vi "JKI_Controller.vi"() -> ()   [LabVIEW 2017, in "Controller_JKI.lvlib"]
uses:
  Controller_JKI.lvlib
  Transaction.ctl
  <userlib>/_NEVSTOP/JKI State Machine ++/_Support/_Create Data Queue.vi
  <userlib>/_NEVSTOP/JKI State Machine ++/_Support/_JKISMQFGV.vi
  <userlib>/_OpenG.lib/array/array.llb/Search 1D Array (String)__ogtk.vi
  <userlib>/_NEVSTOP/JKI State Machine ++/JKI-State-Machine-Plus.lvlib
panel:
  in  "Log In Init Simulator":bool
  out "State History":string
  in  "Name(\"\" to use uuid)":string="Controller"
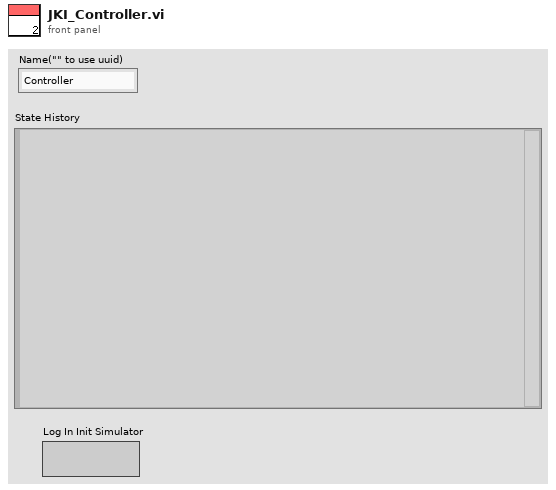
[diagram p1: front panel]
types:
  T1 = typedef "Controller_JKI.lvlib/Transaction.ctl" = enum16{"Welcome", "Login", "Idle ", "Invalid Login", "Terminate Session", "Deposit", "Withdrawl", "Fast Cash", "Withdrawl Complete", "Withdrawl Failed", "Balance Inquiry"}
  T2 = enum32{"Invalid", "Standard", "Closed", "Hidden", "Minimized", "Maximized"}
  T3 = enum32{"invalid app kind", "Development System", "Run Time System", "Student Edition", "Embedded LabVIEW", "Evaluation", "Custom"}
  T4 = cluster{"Core":cluster{"Current VI Reference":refnum<vi>, "Close Panel on Exit?":bool}, "Transactions":T1, "Log in attempts":i32, "First":string, "Last":string, "PIN":string, "Amount":i32, "Money":i32}
  T5 = cluster{"Current VI Reference":refnum<vi>, "Close Panel on Exit?":bool}
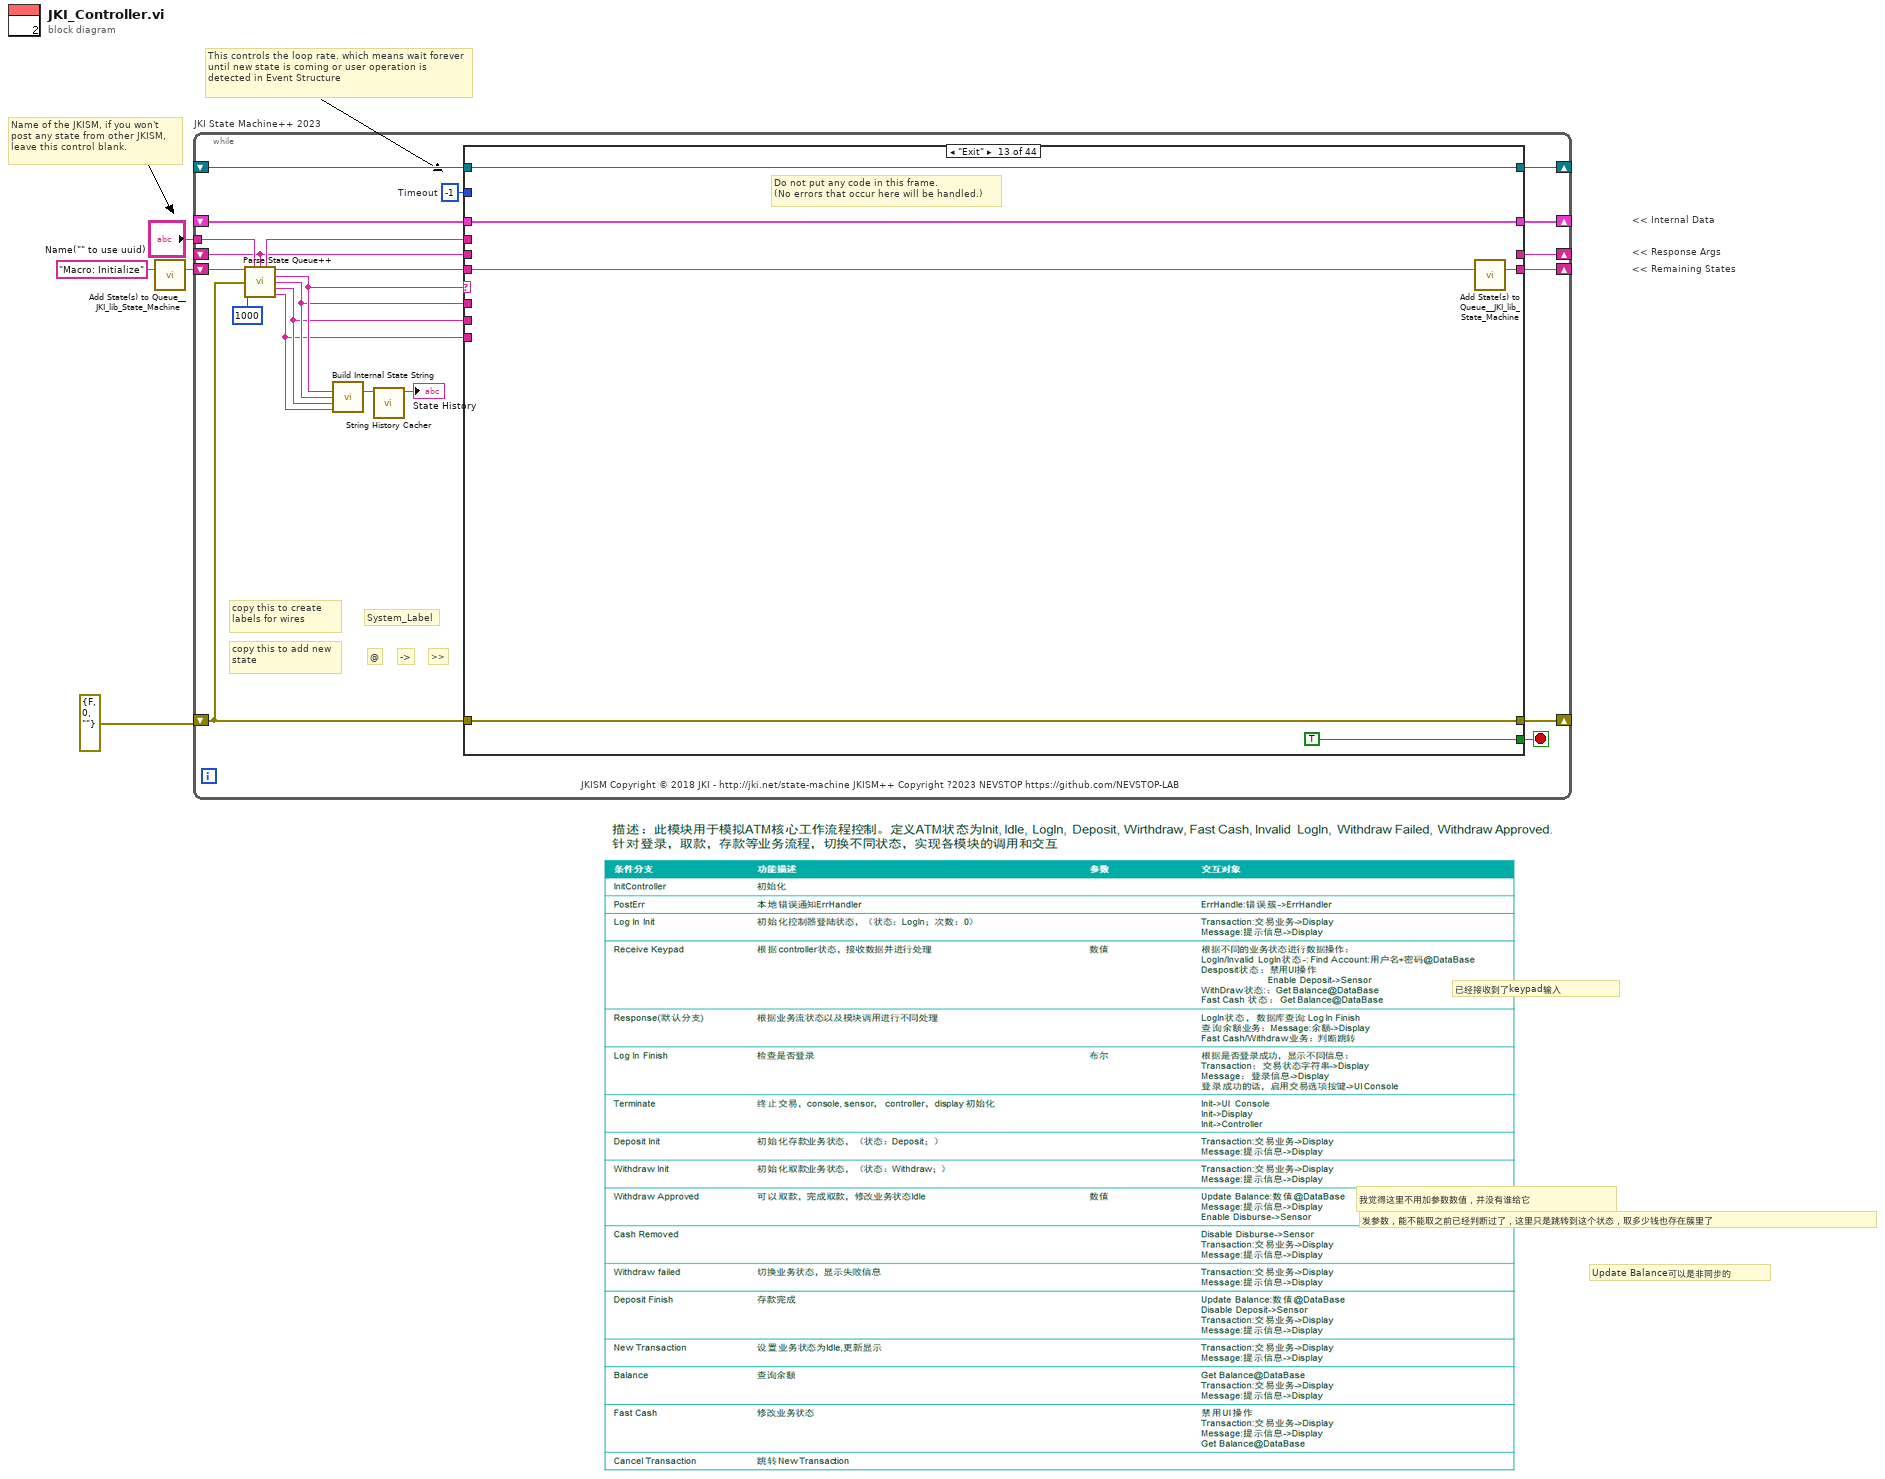
[diagram p0: block diagram]
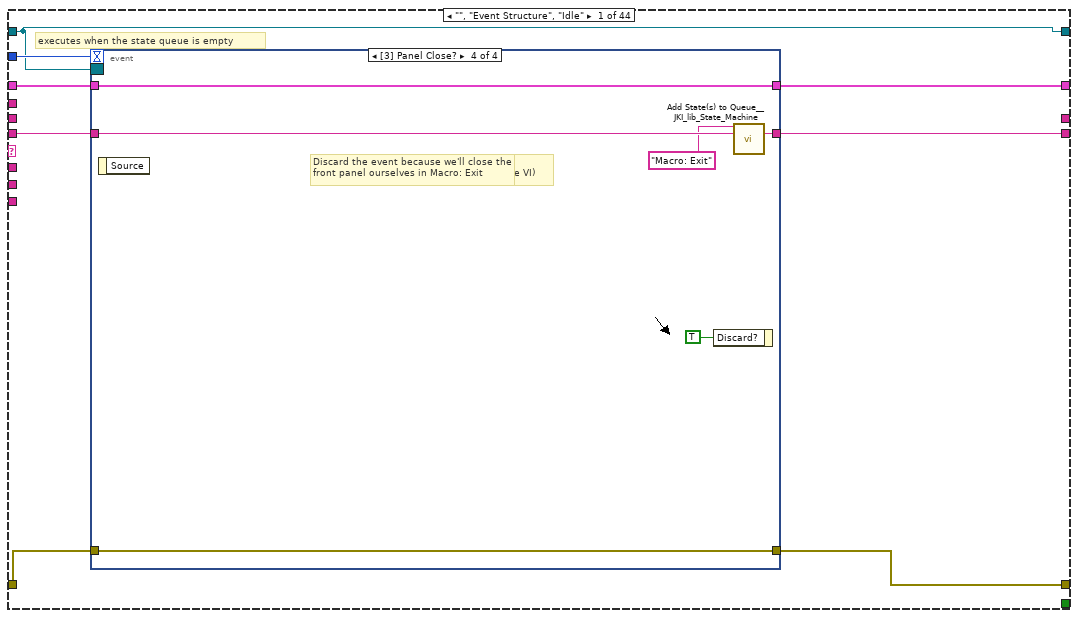
[diagram p2: hidden frame]
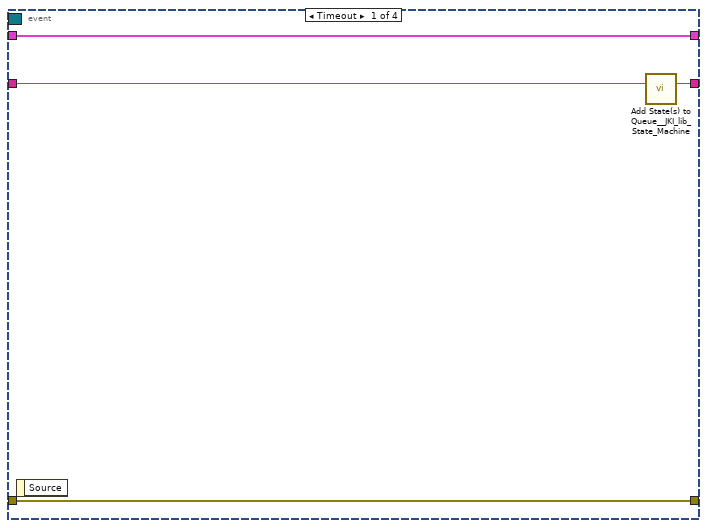
[diagram p3: hidden frame]
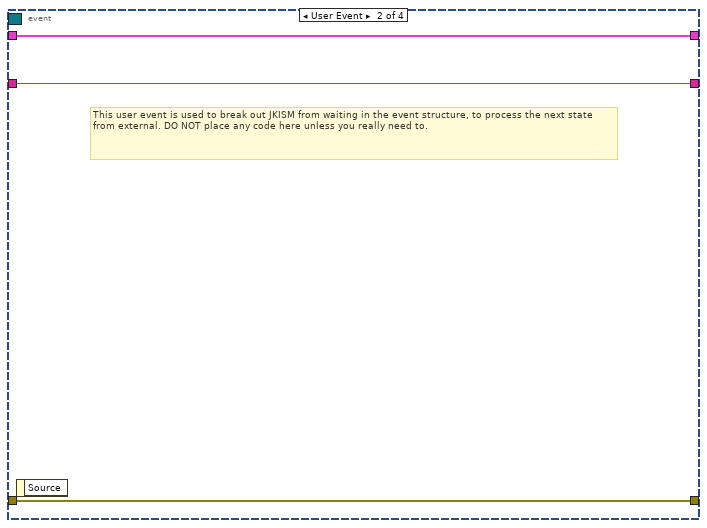
[diagram p4: hidden frame]
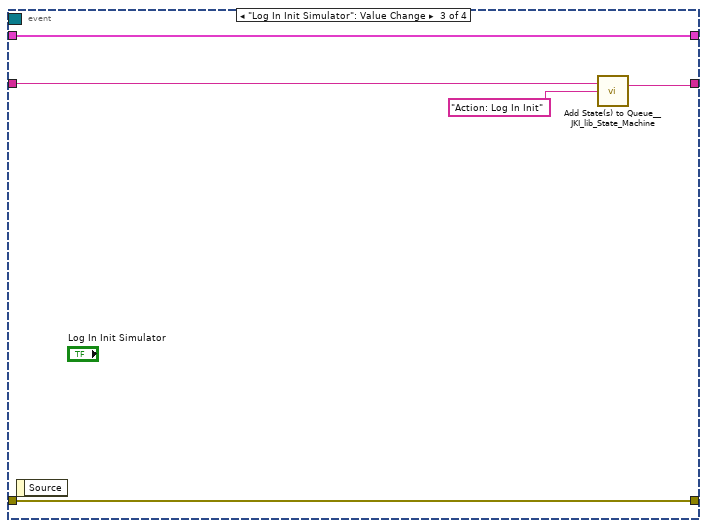
[diagram p5: hidden frame]
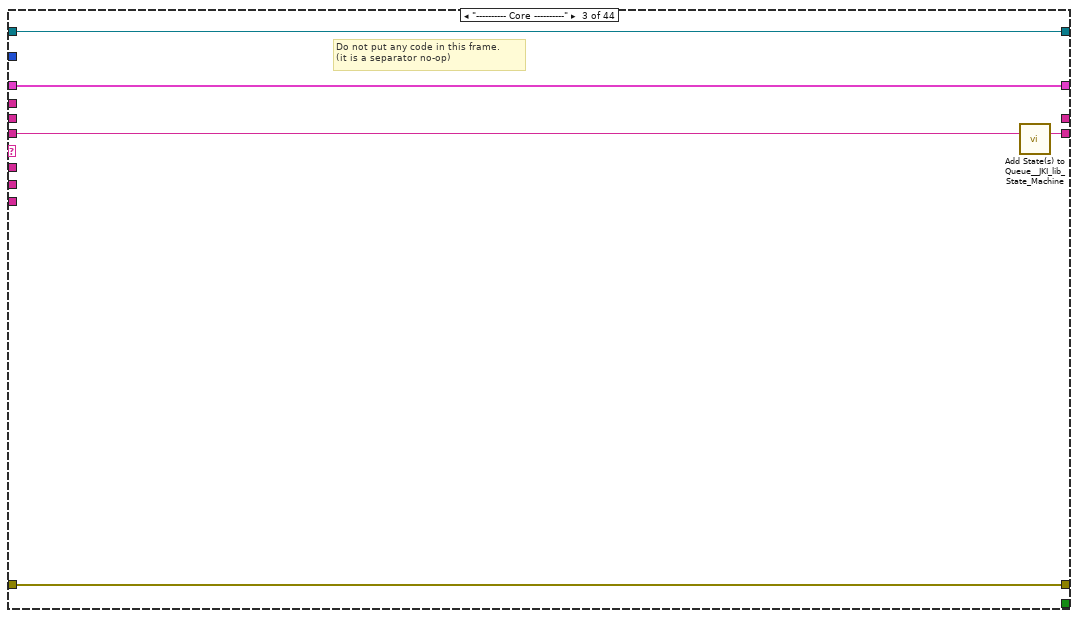
[diagram p7: hidden frame]
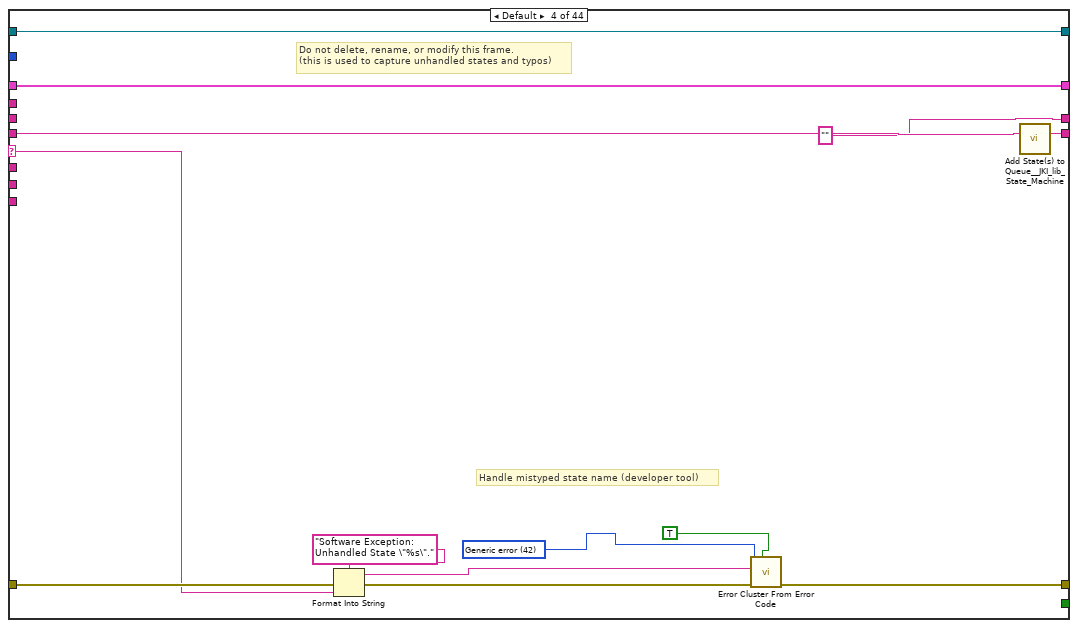
[diagram p8: hidden frame]
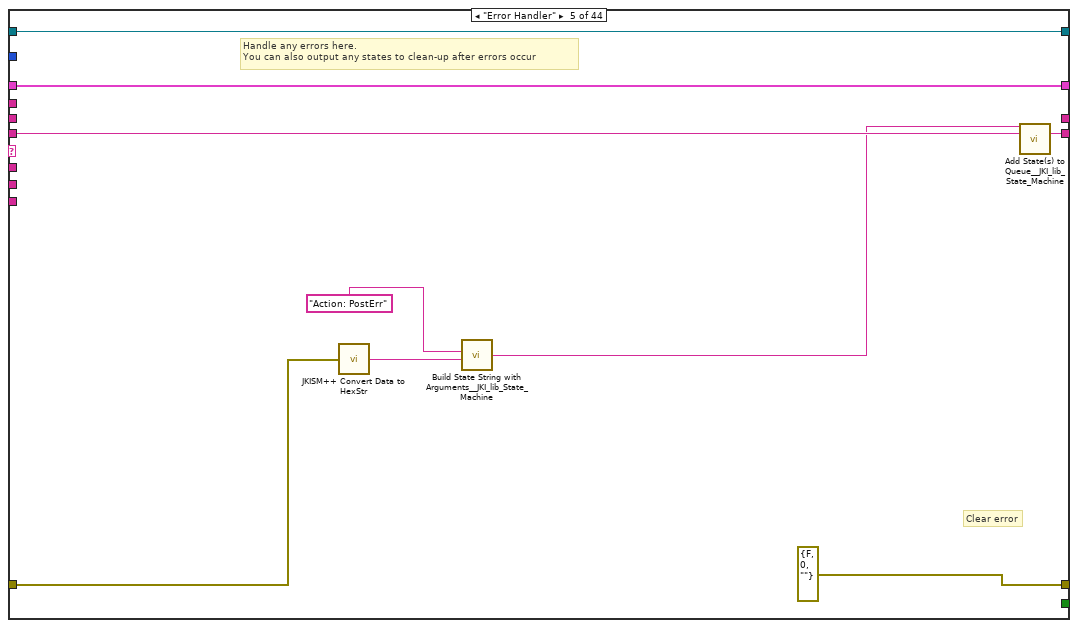
[diagram p9: hidden frame]
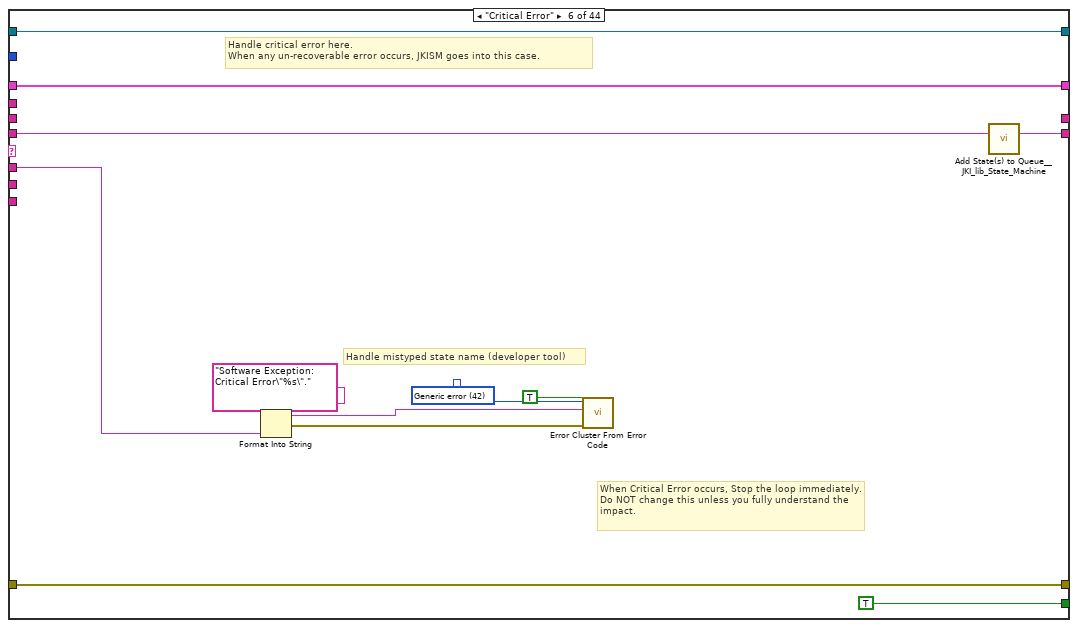
[diagram p10: hidden frame]
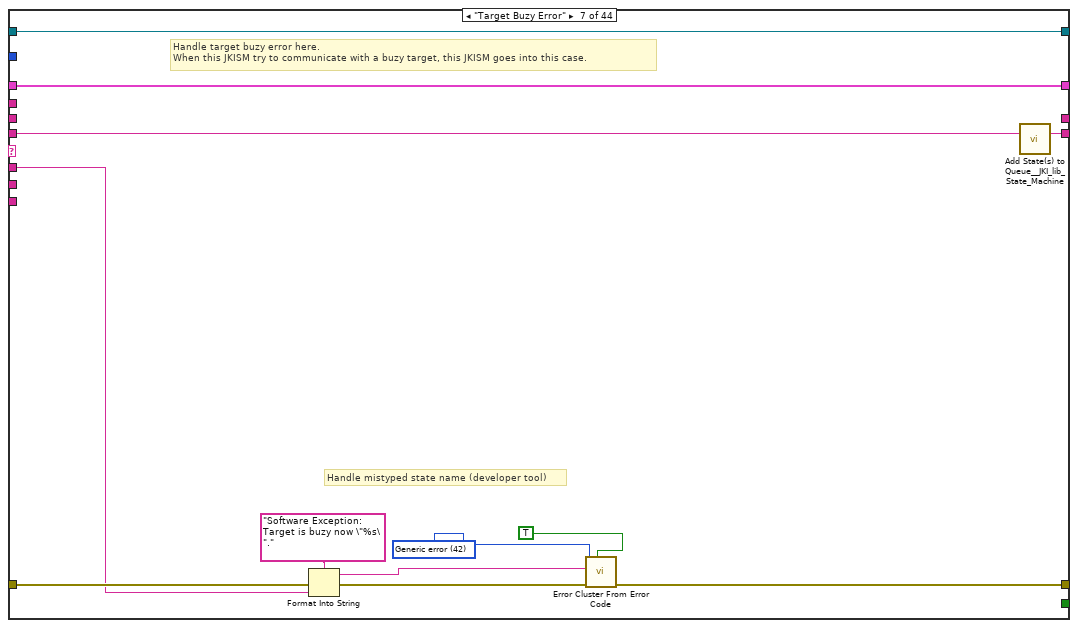
[diagram p11: hidden frame]
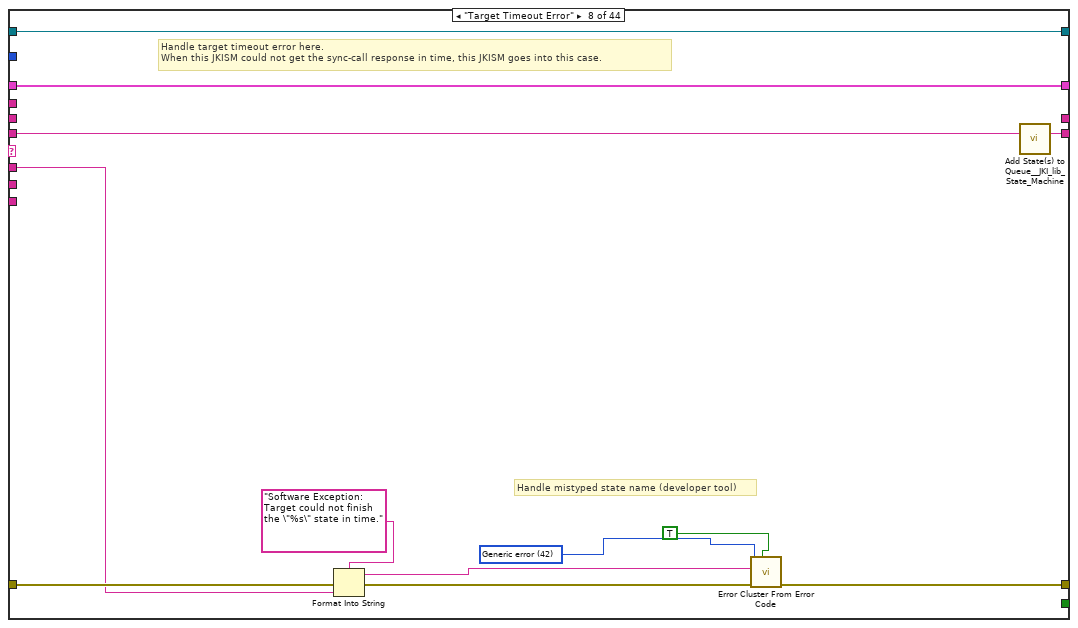
[diagram p12: hidden frame]
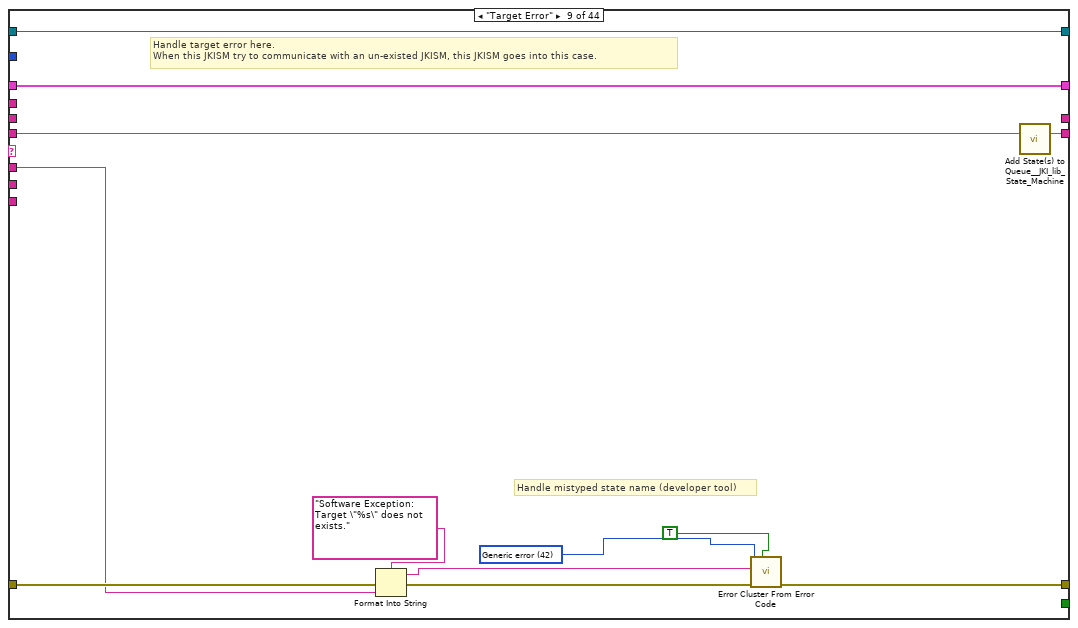
[diagram p13: hidden frame]
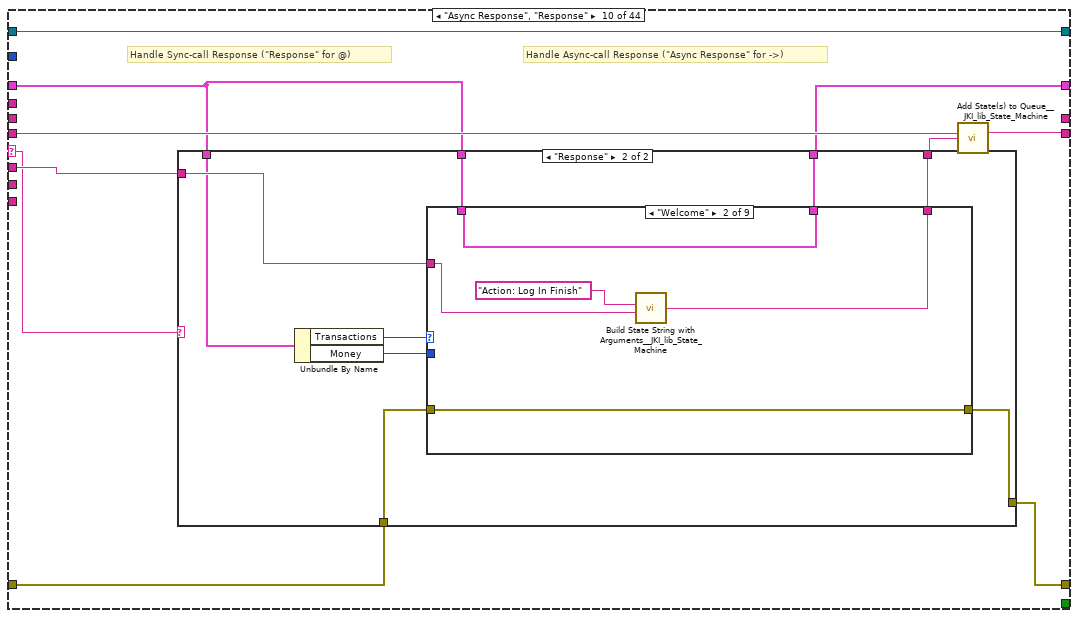
[diagram p14: hidden frame]
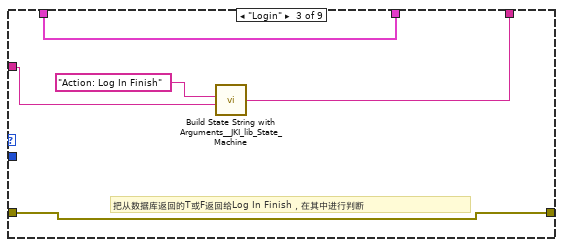
[diagram p17: hidden frame]
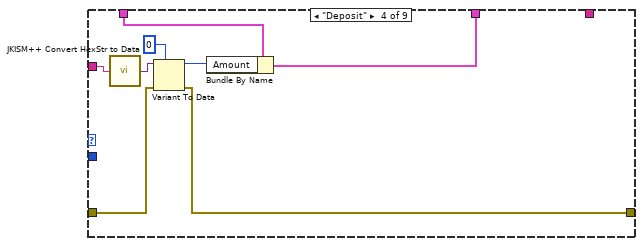
[diagram p18: hidden frame]
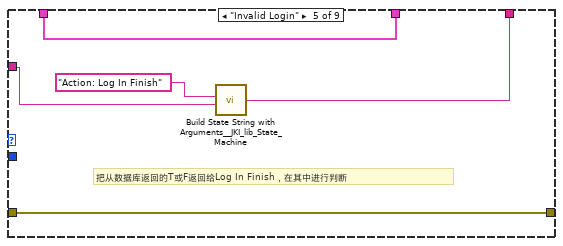
[diagram p19: hidden frame]
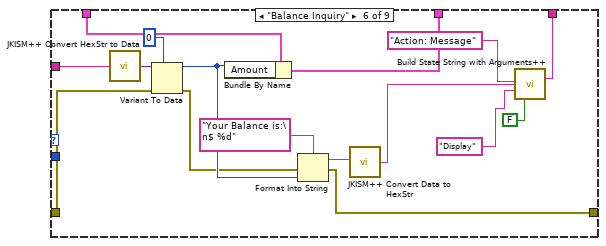
[diagram p20: hidden frame]
diagram:
  # "Update Balance可以是非同步的"
  # "发参数，能不能取之前已经判断过了，这里只是跳转到这个状态，取多少钱也存在簇里了"
  # "我觉得这里不用加参数数值，并没有谁给它"
  # "已经接收到了keypad输入"
  # "<< Internal Data"
  # "<< Response Args"
  # "<< Remaining States"
  # "Name of the JKISM, if you won't post any state from other JKISM,  leave this control blank."
  # "This controls the loop rate. which means wait forever until new state is coming or user operation is detected in Event Structure"
  n1 = call <vilib>:"Add State(s) to Queue__JKI_lib_State_Machine.vi"("State(s) in (\"\")"="Macro: Initialize") -> ("States Out"=w2:string)  [unwired: 14 in]
  n2 = while "JKI State Machine++ 2023" {
    shift-right: [w21] -> _
    shift-left: _ -> [w20]
    shift-right: [w24] -> _
    shift-left: errorcluster {"status"=FALSE, "code"=0, "source"=""} ("error in (no error)") -> [w18]
    shift-right: [w23] -> _
    shift-left: w2 -> [w25]
    tunnel: "Name(\"\" to use uuid)" -> [w13]
    shift-right: [w16] -> _
    shift-left: _ -> [w5]
    shift-right: [w15] -> _
    shift-left: _ -> [w14]
    stop <- w22 stop-if-true
    w19 = -1  # Timeout
    # "JKISM Copyright © 2018 JKI - http://jki.net/state-machine JKISM++ Copyright ?2023 NEVSTOP https://github.com/NEVSTOP-LAB"
    # "copy this to add new state"
    # ">>"
    # "->"
    # "@"
    # "copy this to create labels for wires"
    # "System_Label"
    n3 = call <userlib>:"Parse State Queue++.vi"("State Queue"=w25, "Name(\"\" to use uuid)"=w13, "Response Arguments"=w5, "Error In (no error)"=w18, "Response Timeout(5000ms)"=1000 ("Response Timeout(1000ms)")) -> ("Name Used"=w6:string, "Remaining States"=w26:string, "Current State"=w10:string, "Arguments"=w9:string, "Argument - State"=w8:string, "From Who"=w7:string)  [unwired: 5 in]
    n4 = call <userlib>:"Build Internal State String.vi"("State"=w10, "Arguments (\"\")"=w9, "Arg-State (\"\")"=w8, "Source (\"\")"=w7) -> ("State with Arguments"=w11:string)  [unwired: 11 in]
    n5 = call <userlib>:"String History Cacher.vi"("String"=w11) -> ("String Cache"=→"State History":string)  [unwired: 10 in]
    n6 = case shown="\"Exit\"" w10 {
      selector: w10 -> [_ _ _ w64 _ _ _ _ _ w133 _ _ _ _ _ _ _ _ _ _ _ _ _ _ _ _ _ _ _ _ _ _ _ _ _ _ _ _ _ _ _ _ _ _]
      tunnel: w26 -> [w34 w55 w61 w68 w83 w93 w96 w113 w125 w139 w255 w270 w276 w281 w294 w301 w306 w312 w316 w322 w327 w334 w346 w416 w422 w444 w467 w476 w479 w505 w521 w619 w691 w707 w725 w759 w792 w815 w846 w881 w899 w946 w952 w967]
      tunnel: w9 -> [_ _ _ _ _ w86 w98 w109 w121 w140 _ _ _ _ _ _ _ _ _ _ _ w329 w340 _ _ _ _ _ _ w489 w528 w626 _ _ _ _ _ _ _ _ _ _ _ _]
      tunnel: w20 -> [w32 w54 w58 w66 w80 w94 w100 w111 w123 w132 w254 w263 w274 w278 _ w296 w303 w311 w315 w319 w325 w332 w342 w413 w419 w442 w466 w472 w484 w517 w527 w615 w693 w701 w720 w773 w786 w810 w871 w878 w896 w928 w954 w964]
      tunnel: [w31 w56 w59 w70 errorcluster {"status"=FALSE, "code"=0, "source"=""} ("error out") w95 w103 w115 w127 w135 w256 w267 w273 w279 w291 w297 w304 w307 w314 w320 w324 w330 w343 w414 w420 w427 w468 w474 w485 w497 w522 w616 w679 w704 w723 w740 w796 w813 w830 w876 w894 w919 w961 w965] -> w24
      tunnel: w18 -> [w30 w56 w59 w69 w76 w95 w102 w114 w126 w137 w256 w267 w273 w279 w291 w298 w304 _ w317 w320 w324 w331 w344 w414 w420 w434 w468 w474 w485 w498 w522 w622 w679 w704 w723 w741 w796 w813 w831 w876 w894 w919 w961 w965]
      tunnel: [w33 w55 w60 w67 w82 w92 w101 w112 w124 w138 w255 w269 w275 w280 w293 w300 w305 w312 w316 w321 w326 w333 w345 w415 w421 w443 w467 w475 w478 w504 w520 w618 w690 w706 w726 w758 w791 w816 w845 w880 w898 w945 w951 w966] -> w23
      tunnel: [_ _ _ _ _ TRUE _ _ _ _ _ _ TRUE _ _ _ _ _ _ _ _ _ _ _ _ _ _ _ _ _ _ _ _ _ _ _ _ _ _ _ _ _ _ _] -> w22
      tunnel: [w29 w54 w58 w66 w80 w94 w100 w111 w123 w136 w254 w268 w274 w278 w292 w296 w303 w311 w315 w319 w325 w332 w342 w413 w419 w442 w466 w470 w484 w515 w526 w614 w693 w698 w719 w772 w785 w808 w870 w877 w895 w927 w955 w964] -> w21
      tunnel: w19 -> [w28 _ _ _ _ _ _ _ _ _ _ _ _ _ _ _ _ _ _ _ _ _ _ _ _ _ _ _ _ _ _ _ _ _ _ _ _ _ _ _ _ _ _ _]
      tunnel: w7 -> [_ _ _ _ _ _ _ _ _ _ _ _ _ _ _ _ _ _ _ _ _ _ _ _ _ _ _ _ _ _ _ _ _ _ _ _ _ _ _ _ _ _ _ _]
      tunnel: w8 -> [_ _ _ _ _ _ _ _ _ _ _ _ _ _ _ _ _ _ _ _ _ _ _ _ _ _ _ _ _ _ _ _ _ _ _ _ _ _ _ _ _ _ _ _]
      tunnel: [_ _ _ "" _ _ _ _ _ _ _ _ _ _ _ _ _ _ _ _ _ _ _ _ _ _ _ _ _ _ _ _ _ _ _ _ _ _ _ _ _ _ _ _] -> w16
      tunnel: [w27 w53 w57 w62 w79 w84 w97 w108 w120 w141 w253 w257 w271 w277 w289 w295 w302 w310 w313 w318 w323 w328 w339 w412 w417 w436 w465 w473 w483 w518 w531 w627 w692 w717 w737 w775 w807 w827 w872 w892 w910 w949 w960 w963] -> w15
      tunnel: w14 -> [w27 w53 w57 w62 w79 w84 w97 w108 w120 w141 w253 w257 w271 w277 w289 w295 w302 _ w313 w318 w323 w328 w339 w412 w417 w436 w465 w473 w483 w518 w531 w627 w692 w717 w737 w775 w807 w827 w872 w892 w910 w949 w960 w963]
      tunnel: w6 -> [_ _ _ _ _ _ _ _ _ _ _ _ _ _ _ _ _ w309 _ _ _ _ _ _ _ _ _ _ _ _ _ _ _ _ _ _ _ _ _ _ _ _ _ _]
      tunnel: w5 -> [_ _ _ _ _ _ _ _ _ _ _ _ _ _ _ _ _ _ _ _ _ _ _ _ _ _ _ _ _ _ _ _ _ _ _ _ _ _ _ _ _ _ _ _]
      frame "", "Event Structure", "Idle" {
        # "executes when the state queue is empty"
        n7 = event shown="[3] Panel Close?" {
          selector: w27 -> [_ _ _ _]
          dyn-events: _ -> [_ _ _ _]
          timeout: w28 -> [_ _ _ _]
          tunnel: w34 -> [w38 w40 w44 w52]
          tunnel: [w37 w40 w43 w51] -> w33
          tunnel: w32 -> [w35 w41 w45 w49]
          tunnel: [w36 w39 w46 w50] -> w31
          tunnel: w30 -> [w36 w39 w46 w50]
          tunnel: [w35 w41 w45 w49] -> w29
          event Timeout {
            n8 = event-data() -> ()  [unwired: 1 in, 1 out]
            n9 = call <vilib>:"Add State(s) to Queue__JKI_lib_State_Machine.vi"("State(s) in (\"\")"=w38) -> ("States Out"=w37:string)  [unwired: 14 in]
          }
          event User Event {
            # "This user event is used to break out JKISM from waiting in the event structure, to process the next state from external. DO NOT place any code here unless you really need to."
            n10 = event-data() -> ()  [unwired: 1 in, 1 out]
          }
          event "Log In Init Simulator": Value Change {
            n11 = event-data() -> ()  [unwired: 1 in, 1 out]
            n12 = call <vilib>:"Add State(s) to Queue__JKI_lib_State_Machine.vi"("State(s) in (\"\")"=w44, "State(s) at Back (\"\")"="Action: Log In Init" ("State(s) at Back (\"\")")) -> ("States Out"=w43:string)  [unwired: 13 in]
          }
          event Panel Close? {
            # "Discard the event because we'll close the front panel ourselves in Macro: Exit"
            # "Close Panel button (pressed) Event\n(this executes Macro: Exit to terminate the VI)"
            n13 = event-data() -> ()  [unwired: 1 in, 1 out]
            n14 = event-data("Discard?"=TRUE) -> ()  [unwired: 1 in, 1 out]
            n15 = call <vilib>:"Add State(s) to Queue__JKI_lib_State_Machine.vi"("State(s) in Front (\"\")"="Macro: Exit", "State(s) in (\"\")"=w52) -> ("States Out"=w51:string)  [unwired: 13 in]
          }
        }
      }
      frame "JKISM++ Documentation" {
        # "JKISM++ Documentation"
        # "State Syntax:\nStateCategory: State >> Argument @|-> JKISMName\nLine Terminator: Line feed\n\nExample:\nUI: Help >> About @Main\nUI: Help >> About ->Main"
        # "Commenting:\nTo add a comment use \"//\" or \"#\" and all text to the right will be ignored\nCommenting Example:\nUI: Initialize // This initializes the UI\n# This whole line is a comment\n// Another comment line"
        # "Where \"UI\" is the state category\nWhere \"Help\" is the state\nWhere \"About\" is the argument\nWhere \"Main\" is the Name of JKISM,which actually run the \"UI: Help >> About\"\n\n    \"@\" stands for sync state. Current JKISM will wait until the state is finished. \n            - if \"Main\" named JKISM does not exist, \"Target Error\" will occur.\n            - if \"Main\" named JKISM is in another sync remote state, \"Target Buzy Error\" will occur.\n            - if \"Main\" named JKISM could not finish the state in time, \"Target Timeout Error\" will occur.\n            - if everything is right. \"Response\" will occur with Argument back from \"Main\" named JKISM. \n\n    \"->\" stands for async state. Current JKISM will post the state and continue to next state in next iteration.\n            - if \"Main\" named JKISM does not exist, \"Target Error\" will occur.\n            - if everything is right. \"Async Message Posted\" will occur.\n            - After State is finished. Caller will receive a \"Async Response\" state from callee.\n\nWhen duplicated name is used for multiple JKISM module or some framework problem happens, \"Critical Error\" will occur."
      }
      frame "---------- Core ----------" {
        # "Do not put any code in this frame.\n(it is a separator no-op)"
        n16 = call <vilib>:"Add State(s) to Queue__JKI_lib_State_Machine.vi"("State(s) in (\"\")"=w61) -> ("States Out"=w60:string)  [unwired: 14 in]
      }
      frame Default {
        w73 = 42 items=["No error", "Argument error", "Memory is full", "Out of zone", "End of file", "File already open", "Generic file I/O error", "File not found", "File permission error", "Disk is full", "Duplicate path", "Too many files open", "System feature not enabled", "Resource file not found", "Cannot add resource", "Resource not found", "Image not found", "Image memory error", "Pen does not exist", "Config type invalid", "Config token not found", "Config parse error", "Config memory error", "Bad external code format", "Bad external code offset", "External code not present", "Null window", "Destroy window error", "Null menu", "Print aborted", "Bad print record", "Print driver error", "Windows error during printing", "Memory error during printing", "Print dialog error", "Generic print error", "Invalid device refnum", "Device not found", "Device parameter error", "Device unit error", "Cannot open device", "Device call aborted", "Generic error", "Cancelled by user", "Object ID too low", "Object ID too high", "Object not in heap", "Unknown heap", "Unknown object (invalid DefProc)", "Unknown object (DefProc not in table)", "Message out of range", "Invalid (null) method", "Unknown message", "Manager call not supported", "Bad address", "Network operation in progress", "Network operation timed out", "Connection is busy", "Network attribute not supported", "Network error", "Address in use", "System out of memory", "Connection aborted", "Connection refused", "Not connected", "Already connected", "Connection closed", "Initialization error (interapplication manager)", "Bad occurrence", "Wait on unbound occurrence handler", "Occurrence queue overflow", "Datalog type conflict", "Unused", "Unrecognized type (interapplication manager)", "Memory corrupt", "Failed to make temporary DLL", "Old CIN version", "Drag socket not found", "Failed to load drop-object", "Failed to register OLE object", "Failed to release OLE object", "Format specifier type mismatch", "Unknown format specifier", "Too few format specifiers", "Too many format specifiers", "Scan failed", "Newer CIN version", "Error converting to variant", "Runtime menu error", "Password tampered", "Variant attribute not found", "Incompatible variant data type", "Event data is not available", "Event Store is not present", "Occurrence is not found", "Event Queue is not created", "Event info is not available", "Refnum passed is NULL", "Error retrieving Class GUID", "Error retrieving CoClass GUID", "Error retrieving TypeLib GUID.", "Bad built application magic bytes.", "Specific driver is different from the specific driver associated with the Logical Name.", "There is no session opened to the class driver.", "Max Error", "MAX - Error with config objects", "MAX - Error loading configuration", "MAX - Group not supported"]
        # "Do not delete, rename, or modify this frame.\n(this is used to capture unhandled states and typos)"
        # "Handle mistyped state name (developer tool)"
        n17 = Format Into String(format string="Software Exception: Unhandled State \"%s\"." ("message"), error in=w69, w64) -> (resulting string=w72:string, error out=w71:errorcluster)  [unwired: 1 in]
        n18 = call <vilib>:"Error Cluster From Error Code.vi"("show call chain? (False)"=TRUE, "error in (no error)"=w71, "error message (\"\")"=w72, "error code (0)"=w73) -> ("error out"=w70:errorcluster)  [unwired: 5 in]
        n19 = call <vilib>:"Add State(s) to Queue__JKI_lib_State_Machine.vi"("State(s) in (\"\")"=w68) -> ("States Out"=w67:string)  [unwired: 14 in]
      }
      frame "Error Handler" {
        # "Handle any errors here.\nYou can also output any states to clean-up after errors occur"
        # "Clear error"
        n20 = call <userlib>:"JKISM++ Convert Data to HexStr.vi"("Variant"=w76) -> ("HEX String (0-9,A-F)"=w78:string)  [unwired: 8 in]
        n21 = call <vilib>:"Build State String with Arguments__JKI_lib_State_Machine.vi"("Arguments (\"\")"=w78, "State"="Action: PostErr") -> ("State with Arguments"=w75:string)  [unwired: 4 in]
        n22 = call <vilib>:"Add State(s) to Queue__JKI_lib_State_Machine.vi"("State(s) in Front (\"\")"=w75, "State(s) in (\"\")"=w83) -> ("States Out"=w82:string)  [unwired: 13 in]
      }
      frame "Critical Error" {
        w90 = 42 items=["No error", "Argument error", "Memory is full", "Out of zone", "End of file", "File already open", "Generic file I/O error", "File not found", "File permission error", "Disk is full", "Duplicate path", "Too many files open", "System feature not enabled", "Resource file not found", "Cannot add resource", "Resource not found", "Image not found", "Image memory error", "Pen does not exist", "Config type invalid", "Config token not found", "Config parse error", "Config memory error", "Bad external code format", "Bad external code offset", "External code not present", "Null window", "Destroy window error", "Null menu", "Print aborted", "Bad print record", "Print driver error", "Windows error during printing", "Memory error during printing", "Print dialog error", "Generic print error", "Invalid device refnum", "Device not found", "Device parameter error", "Device unit error", "Cannot open device", "Device call aborted", "Generic error", "Cancelled by user", "Object ID too low", "Object ID too high", "Object not in heap", "Unknown heap", "Unknown object (invalid DefProc)", "Unknown object (DefProc not in table)", "Message out of range", "Invalid (null) method", "Unknown message", "Manager call not supported", "Bad address", "Network operation in progress", "Network operation timed out", "Connection is busy", "Network attribute not supported", "Network error", "Address in use", "System out of memory", "Connection aborted", "Connection refused", "Not connected", "Already connected", "Connection closed", "Initialization error (interapplication manager)", "Bad occurrence", "Wait on unbound occurrence handler", "Occurrence queue overflow", "Datalog type conflict", "Unused", "Unrecognized type (interapplication manager)", "Memory corrupt", "Failed to make temporary DLL", "Old CIN version", "Drag socket not found", "Failed to load drop-object", "Failed to register OLE object", "Failed to release OLE object", "Format specifier type mismatch", "Unknown format specifier", "Too few format specifiers", "Too many format specifiers", "Scan failed", "Newer CIN version", "Error converting to variant", "Runtime menu error", "Password tampered", "Variant attribute not found", "Incompatible variant data type", "Event data is not available", "Event Store is not present", "Occurrence is not found", "Event Queue is not created", "Event info is not available", "Refnum passed is NULL", "Error retrieving Class GUID", "Error retrieving CoClass GUID", "Error retrieving TypeLib GUID.", "Bad built application magic bytes.", "Specific driver is different from the specific driver associated with the Logical Name.", "There is no session opened to the class driver.", "Max Error", "MAX - Error with config objects", "MAX - Error loading configuration", "MAX - Group not supported"]
        # "Handle critical error here.\nWhen any un-recoverable error occurs, JKISM goes into this case."
        # "When Critical Error occurs, Stop the loop immediately. Do NOT change this unless you fully understand the impact."
        # "Handle mistyped state name (developer tool)"
        n23 = Format Into String(format string="Software Exception: Critical Error\"%s\"." ("message"), w86) -> (resulting string=w89:string, error out=w88:errorcluster)  [unwired: 2 in]
        n24 = call <vilib>:"Error Cluster From Error Code.vi"("show call chain? (False)"=TRUE, "error in (no error)"=w88, "error message (\"\")"=w89, "error code (0)"=w90) -> ()  [unwired: 5 in, 1 out]
        n25 = call <vilib>:"Add State(s) to Queue__JKI_lib_State_Machine.vi"("State(s) in (\"\")"=w93) -> ("States Out"=w92:string)  [unwired: 14 in]
      }
      frame "Target Buzy Error" {
        w106 = 42 items=["No error", "Argument error", "Memory is full", "Out of zone", "End of file", "File already open", "Generic file I/O error", "File not found", "File permission error", "Disk is full", "Duplicate path", "Too many files open", "System feature not enabled", "Resource file not found", "Cannot add resource", "Resource not found", "Image not found", "Image memory error", "Pen does not exist", "Config type invalid", "Config token not found", "Config parse error", "Config memory error", "Bad external code format", "Bad external code offset", "External code not present", "Null window", "Destroy window error", "Null menu", "Print aborted", "Bad print record", "Print driver error", "Windows error during printing", "Memory error during printing", "Print dialog error", "Generic print error", "Invalid device refnum", "Device not found", "Device parameter error", "Device unit error", "Cannot open device", "Device call aborted", "Generic error", "Cancelled by user", "Object ID too low", "Object ID too high", "Object not in heap", "Unknown heap", "Unknown object (invalid DefProc)", "Unknown object (DefProc not in table)", "Message out of range", "Invalid (null) method", "Unknown message", "Manager call not supported", "Bad address", "Network operation in progress", "Network operation timed out", "Connection is busy", "Network attribute not supported", "Network error", "Address in use", "System out of memory", "Connection aborted", "Connection refused", "Not connected", "Already connected", "Connection closed", "Initialization error (interapplication manager)", "Bad occurrence", "Wait on unbound occurrence handler", "Occurrence queue overflow", "Datalog type conflict", "Unused", "Unrecognized type (interapplication manager)", "Memory corrupt", "Failed to make temporary DLL", "Old CIN version", "Drag socket not found", "Failed to load drop-object", "Failed to register OLE object", "Failed to release OLE object", "Format specifier type mismatch", "Unknown format specifier", "Too few format specifiers", "Too many format specifiers", "Scan failed", "Newer CIN version", "Error converting to variant", "Runtime menu error", "Password tampered", "Variant attribute not found", "Incompatible variant data type", "Event data is not available", "Event Store is not present", "Occurrence is not found", "Event Queue is not created", "Event info is not available", "Refnum passed is NULL", "Error retrieving Class GUID", "Error retrieving CoClass GUID", "Error retrieving TypeLib GUID.", "Bad built application magic bytes.", "Specific driver is different from the specific driver associated with the Logical Name.", "There is no session opened to the class driver.", "Max Error", "MAX - Error with config objects", "MAX - Error loading configuration", "MAX - Group not supported"]
        # "Handle target buzy error here.\nWhen this JKISM try to communicate with a buzy target, this JKISM goes into this case."
        # "Handle mistyped state name (developer tool)"
        n26 = Format Into String(format string="Software Exception: Target is buzy now \"%s\"." ("message"), error in=w102, w98) -> (resulting string=w105:string, error out=w104:errorcluster)  [unwired: 1 in]
        n27 = call <vilib>:"Error Cluster From Error Code.vi"("show call chain? (False)"=TRUE, "error in (no error)"=w104, "error message (\"\")"=w105, "error code (0)"=w106) -> ("error out"=w103:errorcluster)  [unwired: 5 in]
        n28 = call <vilib>:"Add State(s) to Queue__JKI_lib_State_Machine.vi"("State(s) in (\"\")"=w96) -> ("States Out"=w101:string)  [unwired: 14 in]
      }
      frame "Target Timeout Error" {
        w118 = 42 items=["No error", "Argument error", "Memory is full", "Out of zone", "End of file", "File already open", "Generic file I/O error", "File not found", "File permission error", "Disk is full", "Duplicate path", "Too many files open", "System feature not enabled", "Resource file not found", "Cannot add resource", "Resource not found", "Image not found", "Image memory error", "Pen does not exist", "Config type invalid", "Config token not found", "Config parse error", "Config memory error", "Bad external code format", "Bad external code offset", "External code not present", "Null window", "Destroy window error", "Null menu", "Print aborted", "Bad print record", "Print driver error", "Windows error during printing", "Memory error during printing", "Print dialog error", "Generic print error", "Invalid device refnum", "Device not found", "Device parameter error", "Device unit error", "Cannot open device", "Device call aborted", "Generic error", "Cancelled by user", "Object ID too low", "Object ID too high", "Object not in heap", "Unknown heap", "Unknown object (invalid DefProc)", "Unknown object (DefProc not in table)", "Message out of range", "Invalid (null) method", "Unknown message", "Manager call not supported", "Bad address", "Network operation in progress", "Network operation timed out", "Connection is busy", "Network attribute not supported", "Network error", "Address in use", "System out of memory", "Connection aborted", "Connection refused", "Not connected", "Already connected", "Connection closed", "Initialization error (interapplication manager)", "Bad occurrence", "Wait on unbound occurrence handler", "Occurrence queue overflow", "Datalog type conflict", "Unused", "Unrecognized type (interapplication manager)", "Memory corrupt", "Failed to make temporary DLL", "Old CIN version", "Drag socket not found", "Failed to load drop-object", "Failed to register OLE object", "Failed to release OLE object", "Format specifier type mismatch", "Unknown format specifier", "Too few format specifiers", "Too many format specifiers", "Scan failed", "Newer CIN version", "Error converting to variant", "Runtime menu error", "Password tampered", "Variant attribute not found", "Incompatible variant data type", "Event data is not available", "Event Store is not present", "Occurrence is not found", "Event Queue is not created", "Event info is not available", "Refnum passed is NULL", "Error retrieving Class GUID", "Error retrieving CoClass GUID", "Error retrieving TypeLib GUID.", "Bad built application magic bytes.", "Specific driver is different from the specific driver associated with the Logical Name.", "There is no session opened to the class driver.", "Max Error", "MAX - Error with config objects", "MAX - Error loading configuration", "MAX - Group not supported"]
        # "Handle target timeout error here.\nWhen this JKISM could not get the sync-call response in time, this JKISM goes into this case."
        # "Handle mistyped state name (developer tool)"
        n29 = Format Into String(format string="Software Exception: Target could not finish the \"%s\" state in time." ("message"), error in=w114, w109) -> (resulting string=w117:string, error out=w116:errorcluster)  [unwired: 1 in]
        n30 = call <vilib>:"Error Cluster From Error Code.vi"("show call chain? (False)"=TRUE, "error in (no error)"=w116, "error message (\"\")"=w117, "error code (0)"=w118) -> ("error out"=w115:errorcluster)  [unwired: 5 in]
        n31 = call <vilib>:"Add State(s) to Queue__JKI_lib_State_Machine.vi"("State(s) in (\"\")"=w113) -> ("States Out"=w112:string)  [unwired: 14 in]
      }
      frame "Target Error" {
        w130 = 42 items=["No error", "Argument error", "Memory is full", "Out of zone", "End of file", "File already open", "Generic file I/O error", "File not found", "File permission error", "Disk is full", "Duplicate path", "Too many files open", "System feature not enabled", "Resource file not found", "Cannot add resource", "Resource not found", "Image not found", "Image memory error", "Pen does not exist", "Config type invalid", "Config token not found", "Config parse error", "Config memory error", "Bad external code format", "Bad external code offset", "External code not present", "Null window", "Destroy window error", "Null menu", "Print aborted", "Bad print record", "Print driver error", "Windows error during printing", "Memory error during printing", "Print dialog error", "Generic print error", "Invalid device refnum", "Device not found", "Device parameter error", "Device unit error", "Cannot open device", "Device call aborted", "Generic error", "Cancelled by user", "Object ID too low", "Object ID too high", "Object not in heap", "Unknown heap", "Unknown object (invalid DefProc)", "Unknown object (DefProc not in table)", "Message out of range", "Invalid (null) method", "Unknown message", "Manager call not supported", "Bad address", "Network operation in progress", "Network operation timed out", "Connection is busy", "Network attribute not supported", "Network error", "Address in use", "System out of memory", "Connection aborted", "Connection refused", "Not connected", "Already connected", "Connection closed", "Initialization error (interapplication manager)", "Bad occurrence", "Wait on unbound occurrence handler", "Occurrence queue overflow", "Datalog type conflict", "Unused", "Unrecognized type (interapplication manager)", "Memory corrupt", "Failed to make temporary DLL", "Old CIN version", "Drag socket not found", "Failed to load drop-object", "Failed to register OLE object", "Failed to release OLE object", "Format specifier type mismatch", "Unknown format specifier", "Too few format specifiers", "Too many format specifiers", "Scan failed", "Newer CIN version", "Error converting to variant", "Runtime menu error", "Password tampered", "Variant attribute not found", "Incompatible variant data type", "Event data is not available", "Event Store is not present", "Occurrence is not found", "Event Queue is not created", "Event info is not available", "Refnum passed is NULL", "Error retrieving Class GUID", "Error retrieving CoClass GUID", "Error retrieving TypeLib GUID.", "Bad built application magic bytes.", "Specific driver is different from the specific driver associated with the Logical Name.", "There is no session opened to the class driver.", "Max Error", "MAX - Error with config objects", "MAX - Error loading configuration", "MAX - Group not supported"]
        # "Handle target error here.\nWhen this JKISM try to communicate with an un-existed JKISM, this JKISM goes into this case."
        # "Handle mistyped state name (developer tool)"
        n32 = Format Into String(format string="Software Exception: Target \"%s\" does not exists." ("message"), error in=w126, w121) -> (resulting string=w129:string, error out=w128:errorcluster)  [unwired: 1 in]
        n33 = call <vilib>:"Error Cluster From Error Code.vi"("show call chain? (False)"=TRUE, "error in (no error)"=w128, "error message (\"\")"=w129, "error code (0)"=w130) -> ("error out"=w127:errorcluster)  [unwired: 5 in]
        n34 = call <vilib>:"Add State(s) to Queue__JKI_lib_State_Machine.vi"("State(s) in (\"\")"=w125) -> ("States Out"=w124:string)  [unwired: 14 in]
      }
      frame "Async Response", "Response" {
        # "Handle Async-call Response (\"Async Response\" for ->)"
        # "Handle Sync-call Response (\"Response\" for @)"
        n35 = case shown="\"Response\"" w133 {
          tunnel: w140 -> [_ w151]
          tunnel: w137 -> [w142 w150]
          tunnel: w132 -> [w143 w149]
          tunnel: [w143 w148] -> w136
          tunnel: [w142 w147] -> w135
          tunnel: [_ w145] -> w134
          tunnel: w132 -> [_ w144]
          frame "Async Response", Default {
          }
          frame "Response" {
            n36 = Unbundle By Name(w149) -> ("Transactions"=w152:T1, "Money"=w146:i32)
            n37 = case shown="\"Welcome\"" w152 {
              tunnel: w151 -> [_ w157 w163 w169 w176 w191 w201 w220 w241]
              tunnel: [_ w156 w161 _ w174 w181 w202 w224 w244] -> w145
              tunnel: w150 -> [w153 w155 w160 w167 w173 w184 w198 w223 w234]
              tunnel: w144 -> [w154 w158 w164 w172 w177 w193 w196 w218 w239]
              tunnel: [w154 w158 w164 w171 w177 w192 w195 w217 w238] -> w148
              tunnel: [w153 w155 w160 w166 w173 w182 w197 w223 w233] -> w147
              tunnel: w146 -> [_ _ _ _ _ _ _ w215 w236]
              frame Default {
              }
              frame "Welcome" {
                n38 = call <vilib>:"Build State String with Arguments__JKI_lib_State_Machine.vi"("Arguments (\"\")"=w157, "State"="Action: Log In Finish") -> ("State with Arguments"=w156:string)  [unwired: 4 in]
              }
              frame "Login" {
                # "把从数据库返回的T或F返回给Log In Finish，在其中进行判断"
                n39 = call <vilib>:"Build State String with Arguments__JKI_lib_State_Machine.vi"("Arguments (\"\")"=w163, "State"="Action: Log In Finish") -> ("State with Arguments"=w161:string)  [unwired: 4 in]
              }
              frame "Deposit" {
                n40 = call <userlib>:"JKISM++ Convert HexStr to Data.vi"("HEX String"=w169) -> ("Variant"=w168:variant)  [unwired: 8 in]
                n41 = Variant To Data(error in=w167, type=0, Variant=w168) -> (data=w165:i32, error out=w166:errorcluster)
                n42 = Bundle By Name(cluster=w172, "Amount"=w165) -> (w171:T4)
              }
              frame "Invalid Login" {
                # "把从数据库返回的T或F返回给Log In Finish，在其中进行判断"
                n43 = call <vilib>:"Build State String with Arguments__JKI_lib_State_Machine.vi"("Arguments (\"\")"=w176, "State"="Action: Log In Finish") -> ("State with Arguments"=w174:string)  [unwired: 4 in]
              }
              frame "Balance Inquiry" {
                n44 = call <userlib>:"JKISM++ Convert HexStr to Data.vi"("HEX String"=w191) -> ("Variant"=w190:variant)  [unwired: 8 in]
                n45 = Variant To Data(error in=w184, type=0, Variant=w190) -> (data=w185:i32, error out=w183:errorcluster)
                n46 = Bundle By Name(cluster=w193, "Amount"=w185) -> (w192:T4)
                n47 = Format Into String(format string="Your Balance is:\n$ %d", error in=w183, w185) -> (resulting string=w179:string, error out=w182:errorcluster)  [unwired: 1 in]
                n48 = call <userlib>:"JKISM++ Convert Data to HexStr.vi"("Variant"=w179) -> ("HEX String (0-9,A-F)"=w178:string)  [unwired: 8 in]
                n49 = call <userlib>:"Build State String with Arguments++.vi"("State"="Action: Message" ("States"), "Arguments (\"\")"=w178, "Dest Module (\"\")"="Display" ("Dest Module"), "Sync-Call(@) T By Default/Async-Call(->) F"=FALSE) -> ("State with Arguments"=w181:string)  [unwired: 11 in]
              }
              frame "Fast Cash" {
                n50 = call <userlib>:"JKISM++ Convert HexStr to Data.vi"("HEX String"=w201) -> ("Variant"=w200:variant)  [unwired: 8 in]
                n51 = Variant To Data(error in=w198, type=0 ("y"), Variant=w200) -> (data=w194:i32, error out=w197:errorcluster)
                n52 = Greater Or Equal?(x=w194, y=50) -> (x >= y?=w203:bool)
                n53 = case shown="False" w203 {
                  tunnel: ["Action: Withdraw Failed" "Action: Fast Cash"] -> w202
                  tunnel: w196 -> [w208 w212]
                  tunnel: [w206 w210] -> w195
                  tunnel: w194 -> [_ w211]
                  frame False {
                    # "余额不足即把本次交易额归零"
                    n54 = Bundle By Name(cluster=w208, "Money"=0, "Transactions"=Transaction."Withdrawl Failed") -> (w206:T4)
                  }
                  frame True {
                    n55 = Bundle By Name(cluster=w212, "Amount"=w211) -> (w210:T4)
                  }
                }
              }
              frame "Withdrawl" {
                # "这里是keypad String"
                n56 = call <userlib>:"JKISM++ Convert HexStr to Data.vi"("HEX String"=w220) -> ("Variant"=w222:variant)  [unwired: 8 in]
                n57 = Variant To Data(type=0 ("y"), Variant=w222) -> (data=w216:i32)  [unwired: 1 in, 1 out]
                n58 = Negate(x=w215) -> (-x=w214:i32)
                n59 = Greater Or Equal?(x=w216, y=w214) -> (x >= y?=w219:bool)
                n60 = case shown="True" w219 {
                  tunnel: ["Action: Withdraw Failed" "Action: Withdraw Approved"] -> w224
                  tunnel: w218 -> [w227 w231]
                  tunnel: [w225 w229] -> w217
                  tunnel: w216 -> [_ w230]
                  frame False {
                    n61 = Bundle By Name(cluster=w227, "Money"=0) -> (w225:T4)
                  }
                  frame True {
                    n62 = Bundle By Name(cluster=w231, "Amount"=w230) -> (w229:T4)
                  }
                }
              }
              frame "Withdrawl Failed" {
                # "这里是keypad String"
                n63 = call <userlib>:"JKISM++ Convert HexStr to Data.vi"("HEX String"=w241) -> ("Variant"=w243:variant)  [unwired: 8 in]
                n64 = Variant To Data(error in=w234, type=0 ("y"), Variant=w243) -> (data=w237:i32, error out=w233:errorcluster)
                n65 = Negate(x=w236) -> (-x=w235:i32)
                n66 = Greater Or Equal?(x=w237, y=w235) -> (x >= y?=w240:bool)
                n67 = case shown="True" w240 {
                  tunnel: ["Action: Withdraw Failed" "Action: Withdraw Approved"] -> w244
                  tunnel: w239 -> [w247 w251]
                  tunnel: [w245 w249] -> w238
                  tunnel: w237 -> [_ w250]
                  frame False {
                    n68 = Bundle By Name(cluster=w247, "Money"=0) -> (w245:T4)
                  }
                  frame True {
                    n69 = Bundle By Name(cluster=w251, "Amount"=w250) -> (w249:T4)
                  }
                }
              }
            }
          }
        }
        n70 = call <vilib>:"Add State(s) to Queue__JKI_lib_State_Machine.vi"("State(s) in (\"\")"=w139, "State(s) at Back (\"\")"=w134) -> ("States Out"=w138:string)  [unwired: 13 in]
      }
      frame "Async Message Posted" {
        # "Handle post action for async message (->)."
        # "After Async Message is posted (->), JKISM+ goes to this state for post-action. You can use Argument - State to tell which Async Message is called."
      }
      frame "Initialize Core Data" {
        # "Do not delete, rename, or modify this frame.\n(this is used to determine panel behavior on exit)"
        # "originally closed?"
        # "exe?"
        # "If panel starts closed or is an EXE, then close it when we exit"
        n71 = property class="VI"() -> ("FP.State"=w260:T2)  [unwired: 2 in, 2 out]
        n72 = property class="App"() -> ("App.Kind"=w266:T3)  [unwired: 2 in, 2 out]
        n73 = control-ref of="Current VI Reference"() -> (w261:refnum<vi>)
        n74 = Equal?(x=w260, y=T2."Closed" ("Front Panel Window:State")) -> (x = y?=w258:bool)
        n75 = Equal?(x=w266, y=T3."Run Time System" ("Application:Kind")) -> (x = y?=w264:bool)
        n76 = Or(x=w258, y=w264) -> (x .or. y?=w262:bool)
        n77 = Bundle By Name(cluster=w263, "Core.Current VI Reference"=w261, "Core.Close Panel on Exit?"=w262) -> (w268:T4)
        n78 = call <vilib>:"Add State(s) to Queue__JKI_lib_State_Machine.vi"("State(s) in (\"\")"=w270) -> ("States Out"=w269:string)  [unwired: 14 in]
      }
      frame "Exit" {
        # "Do not put any code in this frame.\n(No errors that occur here will be handled.)"
        n79 = call <vilib>:"Add State(s) to Queue__JKI_lib_State_Machine.vi"("State(s) in (\"\")"=w276) -> ("States Out"=w275:string)  [unwired: 14 in]
      }
      frame "---------- Data ----------" {
        # "Do not put any code in this frame.\n(It is a separator no-op. You can make a copy of this frame to create a new Data frame)"
        n80 = call <vilib>:"Add State(s) to Queue__JKI_lib_State_Machine.vi"("State(s) in (\"\")"=w281) -> ("States Out"=w280:string)  [unwired: 14 in]
      }
      frame "Data: Initialize" {
        w282 = ""  # PIN
        w283 = 0  # Money
        w284 = 0  # Amount
        w285 = ""  # Last
        w286 = ""  # First
        w287 = 0  # Log in attempts
        w290 = T5 {"Current VI Reference"=refnum, "Close Panel on Exit?"=FALSE}  # Core
        # "do not delete - used by framework"
        # "Expand Bundle to add new data elements to shift register data."
        # "Data names and types of shift register data are defined by this bundle."
        # "Initialize the shift-register data, here.\n(data names are defined by what you wire into the bundle function)"
        n81 = Bundle("Core"=w290, "Transactions"=Transaction."Idle ", "Log in attempts"=w287, "First"=w286, "Last"=w285, "PIN"=w282, "Amount"=w284, "Money"=w283) -> (w292:T4)  [unwired: 1 in]
        n82 = call <vilib>:"Add State(s) to Queue__JKI_lib_State_Machine.vi"("State(s) in (\"\")"=w294) -> ("States Out"=w293:string)  [unwired: 14 in]
      }
      frame "Data: Cleanup" {
        # "Cleanup any data and references, here.\n(this is called automatically, by the Macro: Exit)"
        n83 = Unbundle By Name(w296) -> ("Core.Current VI Reference"=w299:refnum<vi>)
        n84 = Close Reference(reference=w299, error in (no error)=w298) -> (error out=w297:errorcluster)
        n85 = call <vilib>:"Add State(s) to Queue__JKI_lib_State_Machine.vi"("State(s) in (\"\")"=w301) -> ("States Out"=w300:string)  [unwired: 14 in]
      }
      frame "---------- Events ----------" {
        # "Do not put any code in this frame.\n(It is a separator no-op. You can make a copy of this frame to create a new UI frame)"
        n86 = call <vilib>:"Add State(s) to Queue__JKI_lib_State_Machine.vi"("State(s) in (\"\")"=w306) -> ("States Out"=w305:string)  [unwired: 14 in]
      }
      frame "Events: Register" {
        # "Register message event to break Waiting in Event structure."
        n87 = call <userlib>:"JKISM++ Get New State Notifier Event.vi"("Name(\"\" to use uuid) in"=w309) -> ("Error out"=w307:errorcluster, "New State Notifier Event"=w308:refnum<user-event>)  [unwired: 9 in]
        n88 = register-events(w308) -> (reference out=w310:refnum<event-registration>)  [unwired: 2 in, 1 out]
      }
      frame "Events: Unregister" {
        n89 = Unregister For Events(event registration refnum=w313, error in=w317) -> (error out=w314:errorcluster)
      }
      frame "---------- UI ----------" {
        # "Do not put any code in this frame.\n(It is a separator no-op. You can make a copy of this frame to create a new UI frame)"
        n90 = call <vilib>:"Add State(s) to Queue__JKI_lib_State_Machine.vi"("State(s) in (\"\")"=w322) -> ("States Out"=w321:string)  [unwired: 14 in]
      }
      frame "UI: Initialize" {
        # "Initialize the User Interface, here.\n(this is called automatically, by the Macro: Init)"
        n91 = call <vilib>:"Add State(s) to Queue__JKI_lib_State_Machine.vi"("State(s) in (\"\")"=w327) -> ("States Out"=w326:string)  [unwired: 14 in]
      }
      frame "UI: Cursor Set" {
        # "Argument"
        # "Set and Unset Cursor Busy.\n(Usage: \"UI: Cursor Set >> Busy|Idle\")"
        n92 = case shown="\"Idle\", Default" w329 {
          tunnel: w331 -> [w336 w338]
          tunnel: [w335 w337] -> w330
          frame "Idle", Default {
            n93 = call <vilib>:"Unset Busy.vi"("error in (no error)"=w336) -> ("error out"=w335:errorcluster)  [unwired: 10 in]
          }
          frame "Busy" {
            n94 = call <vilib>:"Set Busy.vi"("error in (no error)"=w338) -> ("error out"=w337:errorcluster)  [unwired: 9 in, 1 out]
          }
        }
        n95 = call <vilib>:"Add State(s) to Queue__JKI_lib_State_Machine.vi"("State(s) in (\"\")"=w334) -> ("States Out"=w333:string)  [unwired: 14 in]
      }
      frame "UI: Front Panel State" {
        # "Argument"
        # "Set Front Panel Open or Closed\n(Usage: \"UI: Front Panel State >> Open|Close\")"
        n96 = Unbundle By Name(w342) -> ("Core.Current VI Reference"=w341:refnum<vi>)
        n97 = case shown="\"Close\", \"Closed\"" w340 {
          tunnel: w344 -> [w352 w367 w378 w391 w404]
          tunnel: [w354 w368 w380 w393 w406] -> w343
          tunnel: w341 -> [w353 w365 w379 w392 w405]
          frame "Open", "Standard", Default {
            w347 = T2."Standard" ("State")
            n98 = property class="VI"(reference=w353, error in=w352) -> (reference out=w350:refnum<vi>, error out=w351:errorcluster, "FP.State"=w349:T2)
            n99 = Not Equal?(x=w349, y=w347) -> (x != y?=w348:bool)
            n100 = case shown="True" w348 {
              tunnel: [w358 w360] -> w354
              tunnel: w351 -> [w357 w360]
              tunnel: w350 -> [w356 _]
              tunnel: w347 -> [w355 _]
              frame True {
                n101 = invoke class="VI" method="FP.Open"(reference=w356, error in=w357, "Activate"=TRUE, "State"=w355) -> (error out=w358:errorcluster)  [unwired: 1 in, 4 out]
              }
              frame False {
              }
            }
          }
          frame "Close", "Closed" {
            n102 = property class="VI"(reference=w365, error in=w367) -> (reference out=w364:refnum<vi>, error out=w366:errorcluster, "FP.State"=w362:T2)
            n103 = Not Equal?(x=w362, y=T2."Closed" ("Front Panel Window:State")) -> (x != y?=w361:bool)
            n104 = case shown="True" w361 {
              tunnel: [w369 w372] -> w368
              tunnel: w366 -> [w369 w371]
              tunnel: w364 -> [_ w370]
              frame False {
              }
              frame True {
                n105 = invoke class="VI" method="FP.Close"(reference=w370, error in=w371) -> (error out=w372:errorcluster)  [unwired: 1 in, 2 out]
              }
            }
          }
          frame "Hidden", "Hide" {
            w373 = T2."Hidden" ("State")
            n106 = property class="VI"(reference=w379, error in=w378) -> (reference out=w376:refnum<vi>, error out=w377:errorcluster, "FP.State"=w375:T2)
            n107 = Not Equal?(x=w375, y=w373) -> (x != y?=w374:bool)
            n108 = case shown="True" w374 {
              tunnel: [w384 w385] -> w380
              tunnel: w377 -> [w383 w385]
              tunnel: w376 -> [w382 _]
              tunnel: w373 -> [w381 _]
              frame True {
                n109 = invoke class="VI" method="FP.Open"(reference=w382, error in=w383, "State"=w381) -> (error out=w384:errorcluster)  [unwired: 2 in, 4 out]
              }
              frame False {
              }
            }
          }
          frame "Minimize", "Minimized" {
            w386 = T2."Minimized" ("State")
            n110 = property class="VI"(reference=w392, error in=w391) -> (reference out=w389:refnum<vi>, error out=w390:errorcluster, "FP.State"=w388:T2)
            n111 = Not Equal?(x=w388, y=w386) -> (x != y?=w387:bool)
            n112 = case shown="True" w387 {
              tunnel: [w397 w398] -> w393
              tunnel: w390 -> [w396 w398]
              tunnel: w389 -> [w395 _]
              tunnel: w386 -> [w394 _]
              frame True {
                n113 = invoke class="VI" method="FP.Open"(reference=w395, error in=w396, "State"=w394) -> (error out=w397:errorcluster)  [unwired: 2 in, 4 out]
              }
              frame False {
              }
            }
          }
          frame "Maximize", "Maximized" {
            w399 = T2."Maximized" ("State")
            n114 = property class="VI"(reference=w405, error in=w404) -> (reference out=w402:refnum<vi>, error out=w403:errorcluster, "FP.State"=w401:T2)
            n115 = Not Equal?(x=w401, y=w399) -> (x != y?=w400:bool)
            n116 = case shown="True" w400 {
              tunnel: [w410 w411] -> w406
              tunnel: w403 -> [w409 w411]
              tunnel: w402 -> [w408 _]
              tunnel: w399 -> [w407 _]
              frame True {
                n117 = invoke class="VI" method="FP.Open"(reference=w408, error in=w409, "State"=w407) -> (error out=w410:errorcluster)  [unwired: 2 in, 4 out]
              }
              frame False {
              }
            }
          }
        }
        n118 = call <vilib>:"Add State(s) to Queue__JKI_lib_State_Machine.vi"("State(s) in (\"\")"=w346) -> ("States Out"=w345:string)  [unwired: 14 in]
      }
      frame "---------- Macro ----------" {
        # "Do not put any code in this frame.\n(It is a separator no-op. You can make a copy of this frame to create a new Macro frame)"
        n119 = call <vilib>:"Add State(s) to Queue__JKI_lib_State_Machine.vi"("State(s) in (\"\")"=w416) -> ("States Out"=w415:string)  [unwired: 14 in]
      }
      frame "Macro: Initialize" {
        # "Initialization Macro\n(This is called once, when the VI starts)"
        n120 = call <vilib>:"Add State(s) to Queue__JKI_lib_State_Machine.vi"("State(s) in Front (\"\")"="Data: Initialize\nInitialize Core Data\nEvents: Register\nUI: Initialize\nUI: Front Panel State >> Open\nAction: InitController", "State(s) in (\"\")"=w422) -> ("States Out"=w421:string)  [unwired: 13 in]
      }
      frame "Macro: Exit" {
        # "Exit Macro\n(This is called once, when the VI exits)"
        n121 = Unbundle By Name(w442) -> ("Core.Close Panel on Exit?"=w441:bool)
        n122 = for {
          tunnel: string[] ["Database", "Display", "Error Handler", "Sensor", "UI Console"] -> [w460] mode=indexing
          tunnel: w434 -> [w457]
          tunnel: [w456] -> w428 mode=indexing
          tunnel: [w455] -> w424 mode=indexing
          n123 = call <userlib>:"JKISM++ Check If Module Exists.vi"("Error in"=w457, "JKISM Name"=w460) -> ("Error out"=w456:errorcluster, "Exist?"=w459:bool, "JKISM Name(dup)"=w458:string)  [unwired: 7 in]
          n124 = case shown="True" w459 {
            tunnel: w458 -> [_ w462]
            tunnel: [_ w461] -> w455
            frame False {
            }
            frame True {
              n125 = call <userlib>:"Build State String with Arguments++.vi"("State"="Macro: Exit", "Dest Module (\"\")"=w462, "Sync-Call(@) T By Default/Async-Call(->) F"=FALSE) -> ("State with Arguments"=w461:string)  [unwired: 12 in]
            }
          }
        }
        n126 = call-poly <userlib>:"Search Array__ogtk.vi"("Array"=w424, "Element Data"="") -> ("Indices of Elements"=w425:i32[])  [unwired: 7 in]
        n127 = for {
          tunnel: w425 -> [w446] mode=indexing
          shift-right: [w445] -> w423
          shift-left: w424 -> [w447]
          n128 = Delete From Array(array=w447, index=w446) -> (array with subset deleted=w445:string[])  [unwired: 1 in, 1 out]
        }
        n129 = for {
          tunnel: w423 -> [w454] mode=indexing
          shift-right: [w451] -> w432
          shift-left: "" -> [w452]
          shift-right: [w448] -> w427
          shift-left: errorcluster {"status"=FALSE, "code"=0, "source"=""} ("error in (no error)") -> [w450]
          tunnel: w428 -> [w449] mode=indexing
          n130 = Merge Errors(w450, w449) -> (w448:errorcluster)
          n131 = Concatenate Strings(w452, w454, "\r") -> (w451:string)
        }
        n132 = Select(t="UI: Front Panel State >> Close", s=w441, f="") -> (s? t:f=w438:string)
        n133 = Concatenate Strings(w432, "Data: Cleanup\nEvents: Unregister\nExit") -> (w430:string)
        n134 = call <vilib>:"Add State(s) to Queue__JKI_lib_State_Machine.vi"("State(s) in (\"\")"=w438, "State(s) at Back (\"\")"=w430) -> ("States Out"=w437:string)  [unwired: 13 in]
        n135 = call <vilib>:"Add State(s) to Queue__JKI_lib_State_Machine.vi"("State(s) in Front (\"\")"=w437, "State(s) in (\"\")"=w444) -> ("States Out"=w443:string)  [unwired: 13 in]
      }
      frame "---------- Action ----------" {
        # "Do not put any code in this frame.\n(It is a separator no-op. This category is recommanded to use for external API)"
      }
      frame "Action: InitController" {
        # "其实我已经在数据初始化里初始化过了"
        # "Your code here.\n(You can make a copy of, or modify, this frame)"
        n136 = Bundle By Name(cluster=w472, "Transactions"=Transaction."Welcome", "Log in attempts"=0) -> (w470:T4)
        n137 = call <vilib>:"Add State(s) to Queue__JKI_lib_State_Machine.vi"("State(s) in (\"\")"=w476) -> ("States Out"=w475:string)  [unwired: 14 in]
      }
      frame "Action: PostErr" {
        # "Copy/Rename this case for your own API"
        n138 = call <userlib>:"Build State String with Arguments++.vi"("State"="Error Handler", "Dest Module (\"\")"="Error Handler" ("Dest Module (\"\")"), "Sync-Call(@) T By Default/Async-Call(->) F"=FALSE) -> ("State with Arguments"=w477:string)  [unwired: 12 in]
        n139 = call <vilib>:"Add State(s) to Queue__JKI_lib_State_Machine.vi"("State(s) in (\"\")"=w479, "State(s) at Back (\"\")"=w477) -> ("States Out"=w478:string)  [unwired: 13 in]
      }
      frame "Action: Log In Init" {
        w492 = "\r"
        # "用户名会自动读，其他信息都不会"
        # "Copy/Rename this case for your own API"
        n140 = Match Pattern(string=w489, regular expression=",") -> (before substring=w488:string, after substring=w487:string)  [unwired: 1 in, 2 out]
        n141 = Bundle By Name(cluster=w517, "Transactions"=Transaction."Welcome", "Log in attempts"=0, "First"=w488, "Last"=w487, "PIN"="0" ("Last"), "Amount"=0 ("Balance")) -> (w515:T4)
        n142 = Format Into String(format string="Welcome to Acme Bank.\n%s %s\nPlease enter your Account Number on the keypad.\nPress Enter (E) when done.", error in=w498, w488, w487) -> (resulting string=w496:string, error out=w497:errorcluster)  [unwired: 1 in]
        n143 = call <userlib>:"JKISM++ Convert Data to HexStr.vi"("Variant"=w496) -> ("HEX String (0-9,A-F)"=w500:string)  [unwired: 8 in]
        n144 = call <userlib>:"Build State String with Arguments++.vi"("State"="Action: Transaction", "Arguments (\"\")"="Welcome" ("Arguments (\"\")"), "Dest Module (\"\")"="Display" ("Dest Module"), "Sync-Call(@) T By Default/Async-Call(->) F"=FALSE) -> ("State with Arguments"=w507:string)  [unwired: 11 in]
        n145 = call <userlib>:"Build State String with Arguments++.vi"("State"="Action: Enable Keypad", "Dest Module (\"\")"="UI Console" ("Dest Module"), "Sync-Call(@) T By Default/Async-Call(->) F"=FALSE) -> ("State with Arguments"=w491:string)  [unwired: 12 in]
        n146 = call <userlib>:"Build State String with Arguments++.vi"("State"="Action: Message", "Arguments (\"\")"=w500, "Dest Module (\"\")"="Display" ("Dest Module"), "Sync-Call(@) T By Default/Async-Call(->) F"=FALSE) -> ("State with Arguments"=w506:string)  [unwired: 11 in]
        n147 = Concatenate Strings(w507, w492, w506, w492, w491) -> (w503:string)
        n148 = call <vilib>:"Add State(s) to Queue__JKI_lib_State_Machine.vi"("State(s) in (\"\")"=w505, "State(s) at Back (\"\")"=w503) -> ("States Out"=w504:string)  [unwired: 13 in]
      }
      frame "Action: Receive Keypad" {
        # "Keypad输入的密码"
        # "Do not put any code in this frame.\n(It is a separator no-op. This category is recommanded to use for external API)"
        n149 = Unbundle By Name(w527) -> ("Transactions"=w523:T1, "First"=w530:string, "Last"=w529:string, "PIN"=w524:string, "Amount"=w525:i32)  [unwired: 1 out]
        n150 = case shown="\"Deposit\"" w523 {
          tunnel: w530 -> [w536 w549 _ _ _ _ _]
          tunnel: w529 -> [w535 w548 _ _ _ _ _]
          tunnel: w528 -> [w534 w543 w570 w588 w605 _ _]
          tunnel: w527 -> [w537 w551 w571 w587 w604 w612 w613]
          tunnel: [w533 w550 w568 w586 w603 w610 w613] -> w526
          tunnel: w525 -> [_ _ _ _ _ _ _]
          tunnel: w524 -> [_ _ _ w581 w598 w608 _]
          tunnel: [w532 w542 w559 w572 w589 w606 _] -> w519
          frame "Welcome" {
            w541 = ","
            # "用户名+密码去数据库搜"
            n151 = Bundle By Name(cluster=w537, "PIN"=w534) -> (w533:T4)
            n152 = Concatenate Strings(w536, w541, w535, w541, w534) -> (w538:string)
            n153 = call <userlib>:"Build State String with Arguments++.vi"("State"="Action: Find Account" ("States"), "Arguments (\"\")"=w538, "Dest Module (\"\")"="Database" ("Dest Module")) -> ("State with Arguments"=w532:string)  [unwired: 12 in]
          }
          frame "Invalid Login" {
            w547 = ","
            # "用户名+密码去数据库搜"
            n154 = Bundle By Name(cluster=w551, "PIN"=w543) -> (w550:T4)
            n155 = Concatenate Strings(w549, w547, w548, w547, w543) -> (w544:string)
            n156 = call <userlib>:"Build State String with Arguments++.vi"("State"="Action: Find Account" ("States"), "Arguments (\"\")"=w544, "Dest Module (\"\")"="Database" ("Dest Module")) -> ("State with Arguments"=w542:string)  [unwired: 12 in]
          }
          frame "Deposit" {
            w555 = "\r"
            # "暂存本次交易存了多少钱"
            n157 = Decimal String To Number(string=w570) -> (number=w569:i32)  [unwired: 2 in, 1 out]
            n158 = Bundle By Name(cluster=w571, "Money"=w569) -> (w568:T4)
            n159 = call <userlib>:"JKISM++ Convert Data to HexStr.vi"("Variant"="Deposit processing." ("Arguments (\"\")")) -> ("HEX String (0-9,A-F)"=w552:string)  [unwired: 8 in]
            n160 = call <userlib>:"Build State String with Arguments++.vi"("State"="Action: Message" ("Dest Module"), "Arguments (\"\")"=w552, "Dest Module (\"\")"="Display" ("Dest Module"), "Sync-Call(@) T By Default/Async-Call(->) F"=FALSE) -> ("State with Arguments"=w554:string)  [unwired: 11 in]
            n161 = call <userlib>:"Build State String with Arguments++.vi"("State"="Action: Enable Deposit" ("Dest Module"), "Dest Module (\"\")"="Sensor" ("Dest Module"), "Sync-Call(@) T By Default/Async-Call(->) F"=FALSE) -> ("State with Arguments"=w560:string)  [unwired: 12 in]
            n162 = call <userlib>:"Build State String with Arguments++.vi"("State"="Action: InitConsole", "Dest Module (\"\")"="UI Console" ("Dest Module"), "Sync-Call(@) T By Default/Async-Call(->) F"=FALSE) -> ("State with Arguments"=w561:string)  [unwired: 12 in]
            n163 = Concatenate Strings(w561, w555, w560, w555, w554) -> (w559:string)
          }
          frame "Withdrawl" {
            # "暂存本次交易取了多少钱"
            n164 = Decimal String To Number(string=w588) -> (number=w585:i32)  [unwired: 2 in, 1 out]
            n165 = Negate(x=w585) -> (-x=w584:i32)
            n166 = Bundle By Name(cluster=w587, "Money"=w584) -> (w586:T4)
            n167 = call <userlib>:"JKISM++ Convert Data to HexStr.vi"("Variant"="Withdrawl processing." ("Arguments (\"\")")) -> ("HEX String (0-9,A-F)"=w576:string)  [unwired: 8 in]
            n168 = call <userlib>:"Build State String with Arguments++.vi"("State"="Action: Message" ("Dest Module"), "Arguments (\"\")"=w576, "Dest Module (\"\")"="Display" ("Dest Module"), "Sync-Call(@) T By Default/Async-Call(->) F"=FALSE) -> ("State with Arguments"=w573:string)  [unwired: 11 in]
            n169 = call <userlib>:"Build State String with Arguments++.vi"("State"="Action: Get Balance" ("States"), "Arguments (\"\")"=w581, "Dest Module (\"\")"="Database" ("Dest Module")) -> ("State with Arguments"=w574:string)  [unwired: 12 in]
            n170 = Concatenate Strings(w574, "\r", w573) -> (w572:string)
          }
          frame "Withdrawl Failed" {
            # "暂存本次交易取了多少钱"
            n171 = Decimal String To Number(string=w605) -> (number=w602:i32)  [unwired: 2 in, 1 out]
            n172 = Negate(x=w602) -> (-x=w601:i32)
            n173 = Bundle By Name(cluster=w604, "Money"=w601) -> (w603:T4)
            n174 = call <userlib>:"JKISM++ Convert Data to HexStr.vi"("Variant"="Deposit processing." ("Arguments (\"\")")) -> ("HEX String (0-9,A-F)"=w593:string)  [unwired: 8 in]
            n175 = call <userlib>:"Build State String with Arguments++.vi"("State"="Action: Message" ("Dest Module"), "Arguments (\"\")"=w593, "Dest Module (\"\")"="Display" ("Dest Module"), "Sync-Call(@) T By Default/Async-Call(->) F"=FALSE) -> ("State with Arguments"=w590:string)  [unwired: 11 in]
            n176 = call <userlib>:"Build State String with Arguments++.vi"("State"="Action: Get Balance" ("States"), "Arguments (\"\")"=w598, "Dest Module (\"\")"="Database" ("Dest Module")) -> ("State with Arguments"=w591:string)  [unwired: 12 in]
            n177 = Concatenate Strings(w591, "\r", w590) -> (w589:string)
          }
          frame "Fast Cash" {
            n178 = Bundle By Name(cluster=w612, "Money"=-50) -> (w610:T4)
            n179 = call <userlib>:"Build State String with Arguments++.vi"("State"="Action: Get Balance" ("States"), "Arguments (\"\")"=w608, "Dest Module (\"\")"="Database" ("Dest Module")) -> ("State with Arguments"=w606:string)  [unwired: 12 in]
          }
          frame Default {
          }
        }
        n180 = call <vilib>:"Add State(s) to Queue__JKI_lib_State_Machine.vi"("State(s) in (\"\")"=w521, "State(s) at Back (\"\")"=w519) -> ("States Out"=w520:string)  [unwired: 13 in]
      }
      frame "Action: Log In Finish" {
        # "Do not put any code in this frame.\n(It is a separator no-op. This category is recommanded to use for external API)"
        n181 = Unbundle By Name(w615) -> ("First"=w621:string, "Last"=w620:string)
        n182 = call <userlib>:"JKISM++ Convert HexStr to Data.vi"("HEX String"=w626) -> ("Variant"=w625:variant)  [unwired: 8 in]
        n183 = Variant To Data(type=TRUE, Variant=w625) -> (data=w623:bool)  [unwired: 1 in, 1 out]
        n184 = case shown="True" w623 {
          tunnel: w622 -> [w640 w654]
          tunnel: [w640 w653] -> w616
          tunnel: w621 -> [_ w668]
          tunnel: w620 -> [_ w667]
          tunnel: [w634 w662] -> w617
          tunnel: w615 -> [w630 w647]
          tunnel: [w629 w646] -> w614
          frame False {
            n185 = Bundle By Name(cluster=w630, "Transactions"=Transaction."Invalid Login") -> (w629:T4)
            n186 = call <userlib>:"JKISM++ Convert Data to HexStr.vi"("Variant"="Account Information Incorrect\nPlease re-enter your Account Number.\nPress Enter (E) when done.") -> ("HEX String (0-9,A-F)"=w631:string)  [unwired: 8 in]
            n187 = call <userlib>:"Build State String with Arguments++.vi"("State"="Action: Message", "Arguments (\"\")"=w631, "Dest Module (\"\")"="Display" ("Dest Module"), "Sync-Call(@) T By Default/Async-Call(->) F"=FALSE) -> ("State with Arguments"=w637:string)  [unwired: 11 in]
            n188 = call <userlib>:"Build State String with Arguments++.vi"("State"="Action: Transaction", "Arguments (\"\")"="Invalid Login" ("Arguments (\"\")"), "Dest Module (\"\")"="Display" ("Dest Module"), "Sync-Call(@) T By Default/Async-Call(->) F"=FALSE) -> ("State with Arguments"=w638:string)  [unwired: 11 in]
            n189 = Concatenate Strings(w638, "\r", w637) -> (w634:string)
          }
          frame True {
            w655 = "\r"
            n190 = Format Into String(format string="Welcome to Acme Bank\n%s %s\nPlease select a transaction by using the buttons." ("Arguments (\"\")"), error in=w654, w668, w667) -> (resulting string=w649:string, error out=w653:errorcluster)  [unwired: 1 in]
            n191 = call <userlib>:"JKISM++ Convert Data to HexStr.vi"("Variant"=w649) -> ("HEX String (0-9,A-F)"=w648:string)  [unwired: 8 in]
            n192 = Bundle By Name(cluster=w647, "Transactions"=Transaction."Login") -> (w646:T4)
            n193 = call <userlib>:"Build State String with Arguments++.vi"("State"="Action: Transaction", "Arguments (\"\")"="Login" ("Arguments (\"\")"), "Dest Module (\"\")"="Display" ("Dest Module"), "Sync-Call(@) T By Default/Async-Call(->) F"=FALSE) -> ("State with Arguments"=w652:string)  [unwired: 11 in]
            n194 = call <userlib>:"Build State String with Arguments++.vi"("State"="Action: Enable Transaction" ("States"), "Dest Module (\"\")"="UI Console" ("Dest Module"), "Sync-Call(@) T By Default/Async-Call(->) F"=FALSE) -> ("State with Arguments"=w650:string)  [unwired: 12 in]
            n195 = call <userlib>:"Build State String with Arguments++.vi"("State"="Action: Message", "Arguments (\"\")"=w648, "Dest Module (\"\")"="Display" ("Dest Module"), "Sync-Call(@) T By Default/Async-Call(->) F"=FALSE) -> ("State with Arguments"=w651:string)  [unwired: 11 in]
            n196 = Concatenate Strings(w652, w655, w651, w655, w650) -> (w662:string)
          }
        }
        n197 = call <vilib>:"Add State(s) to Queue__JKI_lib_State_Machine.vi"("State(s) in (\"\")"=w619, "State(s) at Back (\"\")"=w617) -> ("States Out"=w618:string)  [unwired: 13 in]
      }
      frame "Action: Terminate" {
        w671 = "\r"
        # "Do not put any code in this frame.\n(It is a separator no-op. This category is recommanded to use for external API)"
        n198 = call <userlib>:"Build State String with Arguments++.vi"("State"="Action: Enable Card Reader" ("States"), "Dest Module (\"\")"="UI Console" ("Dest Module"), "Sync-Call(@) T By Default/Async-Call(->) F"=FALSE) -> ("State with Arguments"=w670:string)  [unwired: 12 in]
        n199 = call <userlib>:"Build State String with Arguments++.vi"("State"="Action: Turn Off the Card Reader", "Dest Module (\"\")"="UI Console" ("Dest Module"), "Sync-Call(@) T By Default/Async-Call(->) F"=FALSE) -> ("State with Arguments"=w675:string)  [unwired: 12 in]
        n200 = call <userlib>:"Build State String with Arguments++.vi"("State"="Action: InitConsole" ("States"), "Dest Module (\"\")"="UI Console" ("Dest Module"), "Sync-Call(@) T By Default/Async-Call(->) F"=FALSE) -> ("State with Arguments"=w683:string)  [unwired: 12 in]
        n201 = call <userlib>:"Build State String with Arguments++.vi"("State"="Action: InitDisplay" ("States"), "Dest Module (\"\")"="Display" ("Dest Module"), "Sync-Call(@) T By Default/Async-Call(->) F"=FALSE) -> ("State with Arguments"=w682:string)  [unwired: 12 in]
        n202 = Concatenate Strings(w675, w671, w683, w671, w682, w671, "Action: InitController" ("State(s) in Front (\"\")"), w671, w670) -> (w680:string)
        n203 = call <vilib>:"Add State(s) to Queue__JKI_lib_State_Machine.vi"("State(s) in (\"\")"=w691, "State(s) at Back (\"\")"=w680) -> ("States Out"=w690:string)  [unwired: 13 in]
      }
      frame "Action: Deposit Init" {
        w696 = "\r"
        # "Do not put any code in this frame.\n(It is a separator no-op. This category is recommanded to use for external API)"
        n204 = Bundle By Name(cluster=w701, "Transactions"=Transaction."Deposit") -> (w698:T4)
        n205 = Unbundle By Name(w698) -> ("PIN"=w697:string)
        n206 = call <userlib>:"JKISM++ Convert Data to HexStr.vi"("Variant"="Please enter amount to deposit and press Enter (E) when done." ("Arguments (\"\")")) -> ("HEX String (0-9,A-F)"=w702:string)  [unwired: 8 in]
        n207 = call <userlib>:"Build State String with Arguments++.vi"("State"="Action: Get Balance" ("States"), "Arguments (\"\")"=w697, "Dest Module (\"\")"="Database" ("Dest Module")) -> ("State with Arguments"=w695:string)  [unwired: 12 in]
        n208 = call <userlib>:"Build State String with Arguments++.vi"("State"="Action: Transaction" ("States"), "Arguments (\"\")"="Deposit" ("Arguments (\"\")"), "Dest Module (\"\")"="Display" ("Dest Module"), "Sync-Call(@) T By Default/Async-Call(->) F"=FALSE) -> ("State with Arguments"=w709:string)  [unwired: 11 in]
        n209 = call <userlib>:"Build State String with Arguments++.vi"("State"="Action: Message" ("States"), "Arguments (\"\")"=w702, "Dest Module (\"\")"="Display" ("Dest Module"), "Sync-Call(@) T By Default/Async-Call(->) F"=FALSE) -> ("State with Arguments"=w708:string)  [unwired: 11 in]
        n210 = Concatenate Strings(w709, w696, w708, w696, w695) -> (w705:string)
        n211 = call <vilib>:"Add State(s) to Queue__JKI_lib_State_Machine.vi"("State(s) in (\"\")"=w707, "State(s) at Back (\"\")"=w705) -> ("States Out"=w706:string)  [unwired: 13 in]
      }
      frame "Action: Withdraw Init" {
        # "Do not put any code in this frame.\n(It is a separator no-op. This category is recommanded to use for external API)"
        n212 = Bundle By Name(cluster=w720, "Transactions"=Transaction."Withdrawl") -> (w719:T4)
        n213 = call <userlib>:"JKISM++ Convert Data to HexStr.vi"("Variant"="Please enter amount to withdraw and press Enter (E) when done." ("Arguments (\"\")")) -> ("HEX String (0-9,A-F)"=w721:string)  [unwired: 8 in]
        n214 = call <userlib>:"Build State String with Arguments++.vi"("State"="Action: Transaction" ("States"), "Arguments (\"\")"="Withdrawl" ("Arguments (\"\")"), "Dest Module (\"\")"="Display" ("Dest Module"), "Sync-Call(@) T By Default/Async-Call(->) F"=FALSE) -> ("State with Arguments"=w728:string)  [unwired: 11 in]
        n215 = call <userlib>:"Build State String with Arguments++.vi"("State"="Action: Message" ("States"), "Arguments (\"\")"=w721, "Dest Module (\"\")"="Display" ("Dest Module"), "Sync-Call(@) T By Default/Async-Call(->) F"=FALSE) -> ("State with Arguments"=w729:string)  [unwired: 11 in]
        n216 = Concatenate Strings(w728, "\r", w729) -> (w724:string)
        n217 = call <vilib>:"Add State(s) to Queue__JKI_lib_State_Machine.vi"("State(s) in (\"\")"=w725, "State(s) at Back (\"\")"=w724) -> ("States Out"=w726:string)  [unwired: 13 in]
      }
      frame "Action: Withdraw Approved" {
        w750 = "\r"
        # "Do not put any code in this frame.\n(It is a separator no-op. This category is recommanded to use for external API)"
        n218 = Unbundle By Name(w773) -> ("Amount"=w774:i32, "Money"=w743:i32, "PIN"=w769:string)
        n219 = Negate(x=w743) -> (-x=w742:i32)
        n220 = Add(x=w774, y=w743) -> (x+y=w770:i32)
        n221 = Format Into String(format string="Please remove cash %d from the ATM." ("Arguments (\"\")"), error in=w741, w742) -> (resulting string=w739:string, error out=w740:errorcluster)  [unwired: 1 in]
        n222 = Bundle By Name(cluster=w773, "Amount"=w770, "Money"=0, "Transactions"=Transaction."Withdrawl Complete") -> (w772:T4)
        n223 = Number To Decimal String(number=w770) -> (decimal integer string=w767:string)  [unwired: 1 in]
        n224 = Concatenate Strings(w769, "," ("string"), w767) -> (w765:string)
        n225 = call <userlib>:"JKISM++ Convert Data to HexStr.vi"("Variant"=w739) -> ("HEX String (0-9,A-F)"=w738:string)  [unwired: 8 in]
        n226 = call <userlib>:"Build State String with Arguments++.vi"("State"="Action: Transaction" ("States"), "Arguments (\"\")"="Withdrawl" ("Arguments (\"\")"), "Dest Module (\"\")"="Display" ("Dest Module"), "Sync-Call(@) T By Default/Async-Call(->) F"=FALSE) -> ("State with Arguments"=w752:string)  [unwired: 11 in]
        n227 = call <userlib>:"Build State String with Arguments++.vi"("State"="Action: Update Balance" ("States"), "Arguments (\"\")"=w765, "Dest Module (\"\")"="Database" ("Dest Module (\"\")")) -> ("State with Arguments"=w753:string)  [unwired: 12 in]
        n228 = call <userlib>:"Build State String with Arguments++.vi"("State"="Action: Message" ("States"), "Arguments (\"\")"=w738, "Dest Module (\"\")"="Display" ("Dest Module"), "Sync-Call(@) T By Default/Async-Call(->) F"=FALSE) -> ("State with Arguments"=w751:string)  [unwired: 11 in]
        n229 = call <userlib>:"Build State String with Arguments++.vi"("State"="Action: Enable Disburse" ("States"), "Dest Module (\"\")"="Sensor" ("Dest Module"), "Sync-Call(@) T By Default/Async-Call(->) F"=FALSE) -> ("State with Arguments"=w749:string)  [unwired: 12 in]
        n230 = Concatenate Strings(w753, w750, w752, w750, w751, w750, w749) -> (w757:string)
        n231 = call <vilib>:"Add State(s) to Queue__JKI_lib_State_Machine.vi"("State(s) in (\"\")"=w759, "State(s) at Back (\"\")"=w757) -> ("States Out"=w758:string)  [unwired: 13 in]
      }
      frame "Action: Cash Removed" {
        w778 = "\r"
        # "Do not put any code in this frame.\n(It is a separator no-op. This category is recommanded to use for external API)"
        n232 = Bundle By Name(cluster=w786, "Transactions"=Transaction."Idle ") -> (w785:T4)
        n233 = call <userlib>:"JKISM++ Convert Data to HexStr.vi"("Variant"="Withdrawl finished." ("Arguments (\"\")")) -> ("HEX String (0-9,A-F)"=w788:string)  [unwired: 8 in]
        n234 = call <userlib>:"Build State String with Arguments++.vi"("State"="Action: Enable Keypad", "Dest Module (\"\")"="UI Console" ("Dest Module (\"\")"), "Sync-Call(@) T By Default/Async-Call(->) F"=FALSE) -> ("State with Arguments"=w777:string)  [unwired: 12 in]
        n235 = call <userlib>:"Build State String with Arguments++.vi"("State"="Action: Enable Transaction", "Dest Module (\"\")"="UI Console" ("Dest Module (\"\")"), "Sync-Call(@) T By Default/Async-Call(->) F"=FALSE) -> ("State with Arguments"=w779:string)  [unwired: 12 in]
        n236 = call <userlib>:"Build State String with Arguments++.vi"("State"="Action: Message" ("States"), "Arguments (\"\")"=w788, "Dest Module (\"\")"="Display" ("Dest Module"), "Sync-Call(@) T By Default/Async-Call(->) F"=FALSE) -> ("State with Arguments"=w793:string)  [unwired: 11 in]
        n237 = call <userlib>:"Build State String with Arguments++.vi"("State"="Action: Transaction" ("States"), "Arguments (\"\")"="Idle" ("Arguments (\"\")"), "Dest Module (\"\")"="Display" ("Dest Module"), "Sync-Call(@) T By Default/Async-Call(->) F"=FALSE) -> ("State with Arguments"=w794:string)  [unwired: 11 in]
        n238 = call <userlib>:"Build State String with Arguments++.vi"("State"="Action: Disable Disburse " ("States"), "Dest Module (\"\")"="Sensor" ("Dest Module"), "Sync-Call(@) T By Default/Async-Call(->) F"=FALSE) -> ("State with Arguments"=w795:string)  [unwired: 12 in]
        n239 = Concatenate Strings(w795, w778, w794, w778, w793, w778, w779, w778, w777) -> (w790:string)
        n240 = call <vilib>:"Add State(s) to Queue__JKI_lib_State_Machine.vi"("State(s) in (\"\")"=w792, "State(s) at Back (\"\")"=w790) -> ("States Out"=w791:string)  [unwired: 13 in]
      }
      frame "Action: Withdraw Failed" {
        # "Do not put any code in this frame.\n(It is a separator no-op. This category is recommanded to use for external API)"
        n241 = Bundle By Name(cluster=w810, "Transactions"=Transaction."Withdrawl Failed") -> (w808:T4)
        n242 = call <userlib>:"JKISM++ Convert Data to HexStr.vi"("Variant"="Insufficient funds in account.\nPlease check your account balance and try again." ("Arguments (\"\")")) -> ("HEX String (0-9,A-F)"=w811:string)  [unwired: 8 in]
        n243 = call <userlib>:"Build State String with Arguments++.vi"("State"="Action: Message" ("States"), "Arguments (\"\")"=w811, "Dest Module (\"\")"="Display" ("Dest Module"), "Sync-Call(@) T By Default/Async-Call(->) F"=FALSE) -> ("State with Arguments"=w817:string)  [unwired: 11 in]
        n244 = call <userlib>:"Build State String with Arguments++.vi"("State"="Action: Transaction" ("States"), "Arguments (\"\")"="Withdrawl Failed" ("Arguments (\"\")"), "Dest Module (\"\")"="Display" ("Dest Module"), "Sync-Call(@) T By Default/Async-Call(->) F"=FALSE) -> ("State with Arguments"=w819:string)  [unwired: 11 in]
        n245 = Concatenate Strings(w819, "\r", w817) -> (w814:string)
        n246 = call <vilib>:"Add State(s) to Queue__JKI_lib_State_Machine.vi"("State(s) in (\"\")"=w815, "State(s) at Back (\"\")"=w814) -> ("States Out"=w816:string)  [unwired: 13 in]
      }
      frame "Action: Deposit Finish" {
        w836 = "\r"
        # "Do not put any code in this frame.\n(It is a separator no-op. This category is recommanded to use for external API)"
        n247 = Unbundle By Name(w871) -> ("Amount"=w868:i32, "Money"=w829:i32, "PIN"=w867:string)
        n248 = Add(x=w868, y=w829) -> (x+y=w865:i32)
        n249 = Number To Decimal String(number=w865) -> (decimal integer string=w864:string)  [unwired: 1 in]
        n250 = Bundle By Name(cluster=w871, "Amount"=w865, "Money"=0) -> (w870:T4)
        n251 = Concatenate Strings(w867, "," ("string"), w864) -> (w863:string)
        n252 = Format Into String(format string="You just deposited %d. " ("Arguments (\"\")"), error in=w831, w829) -> (resulting string=w828:string, error out=w830:errorcluster)  [unwired: 1 in]
        n253 = call <userlib>:"JKISM++ Convert Data to HexStr.vi"("Variant"=w828) -> ("HEX String (0-9,A-F)"=w843:string)  [unwired: 8 in]
        n254 = call <userlib>:"Build State String with Arguments++.vi"("State"="Action: Enable Keypad", "Dest Module (\"\")"="UI Console" ("Dest Module (\"\")"), "Sync-Call(@) T By Default/Async-Call(->) F"=FALSE) -> ("State with Arguments"=w834:string)  [unwired: 12 in]
        n255 = call <userlib>:"Build State String with Arguments++.vi"("State"="Action: Message" ("States"), "Arguments (\"\")"=w843, "Dest Module (\"\")"="Display" ("Dest Module"), "Sync-Call(@) T By Default/Async-Call(->) F"=FALSE) -> ("State with Arguments"=w847:string)  [unwired: 11 in]
        n256 = call <userlib>:"Build State String with Arguments++.vi"("State"="Action: Enable Transaction", "Dest Module (\"\")"="UI Console" ("Dest Module (\"\")"), "Sync-Call(@) T By Default/Async-Call(->) F"=FALSE) -> ("State with Arguments"=w835:string)  [unwired: 12 in]
        n257 = call <userlib>:"Build State String with Arguments++.vi"("State"="Action: Disable Deposit" ("States"), "Dest Module (\"\")"="Sensor" ("Dest Module"), "Sync-Call(@) T By Default/Async-Call(->) F"=FALSE) -> ("State with Arguments"=w849:string)  [unwired: 12 in]
        n258 = call <userlib>:"Build State String with Arguments++.vi"("State"="Action: Transaction" ("States"), "Arguments (\"\")"="Idle" ("Arguments (\"\")"), "Dest Module (\"\")"="Display" ("Dest Module"), "Sync-Call(@) T By Default/Async-Call(->) F"=FALSE) -> ("State with Arguments"=w848:string)  [unwired: 11 in]
        n259 = call <userlib>:"Build State String with Arguments++.vi"("State"="Action: Update Balance" ("States"), "Arguments (\"\")"=w863, "Dest Module (\"\")"="Database" ("Dest Module"), "Sync-Call(@) T By Default/Async-Call(->) F"=FALSE) -> ("State with Arguments"=w851:string)  [unwired: 11 in]
        n260 = Concatenate Strings(w851, w836, w849, w836, w848, w836, w847, w836, w835, w836, w834) -> (w844:string)
        n261 = call <vilib>:"Add State(s) to Queue__JKI_lib_State_Machine.vi"("State(s) in (\"\")"=w846, "State(s) at Back (\"\")"=w844) -> ("States Out"=w845:string)  [unwired: 13 in]
      }
      frame "Action: New Transaction" {
        # "Do not put any code in this frame.\n(It is a separator no-op. This category is recommanded to use for external API)"
        n262 = Bundle By Name(cluster=w878, "Transactions"=Transaction."Idle ") -> (w877:T4)
        n263 = call <userlib>:"JKISM++ Convert Data to HexStr.vi"("Variant"="Please select a transaction by using the buttons." ("Arguments (\"\")")) -> ("HEX String (0-9,A-F)"=w873:string)  [unwired: 8 in]
        n264 = call <userlib>:"Build State String with Arguments++.vi"("State"="Action: Message" ("States"), "Arguments (\"\")"=w873, "Dest Module (\"\")"="Display" ("Dest Module"), "Sync-Call(@) T By Default/Async-Call(->) F"=FALSE) -> ("State with Arguments"=w883:string)  [unwired: 11 in]
        n265 = call <userlib>:"Build State String with Arguments++.vi"("State"="Action: Transaction" ("States"), "Arguments (\"\")"="Idle" ("Arguments (\"\")"), "Dest Module (\"\")"="Display" ("Dest Module"), "Sync-Call(@) T By Default/Async-Call(->) F"=FALSE) -> ("State with Arguments"=w884:string)  [unwired: 11 in]
        n266 = Concatenate Strings(w884, "\r", w883) -> (w879:string)
        n267 = call <vilib>:"Add State(s) to Queue__JKI_lib_State_Machine.vi"("State(s) in (\"\")"=w881, "State(s) at Back (\"\")"=w879) -> ("States Out"=w880:string)  [unwired: 13 in]
      }
      frame "Action: Balance" {
        # "Do not put any code in this frame.\n(It is a separator no-op. This category is recommanded to use for external API)"
        n268 = Unbundle By Name(w896) -> ("PIN"=w904:string)
        n269 = call <userlib>:"Build State String with Arguments++.vi"("State"="Action: Get Balance" ("States"), "Arguments (\"\")"=w904, "Dest Module (\"\")"="Database" ("Dest Module")) -> ("State with Arguments"=w902:string)  [unwired: 12 in]
        n270 = call <userlib>:"Build State String with Arguments++.vi"("State"="Action: Transaction" ("States"), "Arguments (\"\")"="Balance Inquiry" ("Arguments (\"\")"), "Dest Module (\"\")"="Display" ("Dest Module"), "Sync-Call(@) T By Default/Async-Call(->) F"=FALSE) -> ("State with Arguments"=w901:string)  [unwired: 11 in]
        n271 = Bundle By Name(cluster=w896, "Transactions"=Transaction."Balance Inquiry") -> (w895:T4)
        n272 = Concatenate Strings(w902, "\r", w901) -> (w897:string)
        n273 = call <vilib>:"Add State(s) to Queue__JKI_lib_State_Machine.vi"("State(s) in (\"\")"=w899, "State(s) at Back (\"\")"=w897) -> ("States Out"=w898:string)  [unwired: 13 in]
      }
      frame "Action: Fast Cash" {
        w916 = "\r"
        # "Do not put any code in this frame.\n(It is a separator no-op. This category is recommanded to use for external API)"
        n274 = Unbundle By Name(w928) -> ("Amount"=w920:i32, "Money"=w934:i32, "PIN"=w931:string)
        n275 = Add(x=w920, y=w934) -> (x+y=w932:i32)
        n276 = Number To Decimal String(number=w932) -> (decimal integer string=w929:string)  [unwired: 1 in]
        n277 = Bundle By Name(cluster=w928, "Amount"=w932, "Money"=0) -> (w927:T4)
        n278 = Concatenate Strings(w931, "," ("string"), w929) -> (w926:string)
        n279 = call <userlib>:"JKISM++ Convert Data to HexStr.vi"("Variant"="Please take your Fast Cash $50." ("Arguments (\"\")")) -> ("HEX String (0-9,A-F)"=w913:string)  [unwired: 8 in]
        n280 = call <userlib>:"Build State String with Arguments++.vi"("State"="Action: Enable Disburse" ("States"), "Dest Module (\"\")"="Sensor" ("Dest Module (\"\")"), "Sync-Call(@) T By Default/Async-Call(->) F"=FALSE) -> ("State with Arguments"=w915:string)  [unwired: 12 in]
        n281 = call <userlib>:"Build State String with Arguments++.vi"("State"="Action: Update Balance" ("States"), "Arguments (\"\")"=w926, "Dest Module (\"\")"="Database" ("Dest Module (\"\")"), "Sync-Call(@) T By Default/Async-Call(->) F"=FALSE) -> ("State with Arguments"=w922:string)  [unwired: 11 in]
        n282 = call <userlib>:"Build State String with Arguments++.vi"("State"="Action: InitConsole", "Dest Module (\"\")"="UI Console" ("Dest Module"), "Sync-Call(@) T By Default/Async-Call(->) F"=FALSE) -> ("State with Arguments"=w925:string)  [unwired: 12 in]
        n283 = call <userlib>:"Build State String with Arguments++.vi"("State"="Action: Transaction" ("States"), "Arguments (\"\")"="Fast Cash" ("Arguments (\"\")"), "Dest Module (\"\")"="Display" ("Dest Module"), "Sync-Call(@) T By Default/Async-Call(->) F"=FALSE) -> ("State with Arguments"=w924:string)  [unwired: 11 in]
        n284 = call <userlib>:"Build State String with Arguments++.vi"("State"="Action: Message" ("States"), "Arguments (\"\")"=w913, "Dest Module (\"\")"="Display" ("Dest Module"), "Sync-Call(@) T By Default/Async-Call(->) F"=FALSE) -> ("State with Arguments"=w923:string)  [unwired: 11 in]
        n285 = Concatenate Strings(w925, w916, w924, w916, w923, w916, w922, w916, w915) -> (w921:string)
        n286 = call <vilib>:"Add State(s) to Queue__JKI_lib_State_Machine.vi"("State(s) in (\"\")"=w946, "State(s) at Back (\"\")"=w921) -> ("States Out"=w945:string)  [unwired: 13 in]
      }
      frame "Action: Fast Cash Enough" {
        # "Do not put any code in this frame.\n(It is a separator no-op. This category is recommanded to use for external API)"
        n287 = Unbundle By Name(w954) -> ("PIN"=w953:string)
        n288 = Bundle By Name(cluster=w954, "Transactions"=Transaction."Fast Cash", "Money"=-50) -> (w955:T4)
        n289 = call <userlib>:"Build State String with Arguments++.vi"("State"="Action: Get Balance" ("States"), "Arguments (\"\")"=w953, "Dest Module (\"\")"="Database" ("Dest Module")) -> ("State with Arguments"=w950:string)  [unwired: 12 in]
        n290 = call <vilib>:"Add State(s) to Queue__JKI_lib_State_Machine.vi"("State(s) in (\"\")"=w952, "State(s) at Back (\"\")"=w950) -> ("States Out"=w951:string)  [unwired: 13 in]
      }
      frame "Action: Cancel Transaction" {
        # "Your code here.\n(You can make a copy of, or modify, this frame)"
        n291 = call <vilib>:"Add State(s) to Queue__JKI_lib_State_Machine.vi"("State(s) in Front (\"\")"="Action: New Transaction" ("State(s) in Front (\"\")"), "State(s) in (\"\")"=w967) -> ("States Out"=w966:string)  [unwired: 13 in]
      }
    }
  }
